vi "Measurement.vi"(0 "Position":T7(array[cluster]) {"Z" format="%.1f"; "Y" format="%.1f"; "X" format="%.1f"}, 1 "setup":T8=enum."Show Setup", 2 "Post Process":T5, 4 "File":T9, 5 "Results file":path, 7 "Raw data file":path, 11 "Setup filename":string) -> (14 "2nd plot":cluster{"Xo":dbl, "Delta X":dbl, dbl[]}[](graph), 19 "Status Out":T4)   [LabVIEW 2010]
uses:
  Anemometry Sub Vis/Controls/Save_Data.ctl
  Anemometry Sub Vis/Controls/Setup.ctl
  Anemometry Sub Vis/Controls/Graph_Type.ctl
  Anemometry Sub Vis/Controls/Post_Process.ctl
  Anemometry Sub Vis/Gen Trav/Multi_Run_Status.ctl
  Anemometry Sub Vis/Controls/Board_Types.ctl
  Anemometry Sub Vis/Controls/Block_start_and_end.ctl
  ADAM Client/Sub VIs/ADAM Controls/Traverse_Level_State.ctl
  Anemometry Sub Vis/Globals/Trav_pos_global.vi
  Anemometry Sub Vis/Globals/Meas_global.vi
  Anemometry Sub Vis/Acquisition/PWA/PWAtasksGLOBAL.vi
  Anemometry Sub Vis/Globals/Preference_global.vi
  Anemometry Sub Vis/Globals/LDA_meas_global_1.vi
  Anemometry Sub Vis/Globals/Dynamic_call_global.ph.vi
  Anemometry Sub Vis/Globals/LDA_meas_global_2.vi
  Anemometry Sub Vis/Globals/Constants_global.vi
  Anemometry Sub Vis/Globals/Plug_in_data_global.vi
panel:
  in  "PP next block":bool
  out "Pause message":string
  out "Statistics":string[][](table)
  in  "Tab Control":T1(tab)
  out "Measurement time (min)":dbl=6.0 format="%.2f"
  in  "No of bins":i32=80
  in  "Show Smoth":bool=TRUE
  in  "Second Graph":T3={"Plot 1"=2, "Plot 2"=1, "Save graph"=0, "Plot Type"=enum."Vel histogram"} {"Save graph" items=["Do not save plot", "Save plot"]; "Plot 2" items=["Nothing", "LDA (U)", "LDA (W)", "HW (HW) LDA Sync", "HW (HW)", "RV (WT)", "RV (WT2)"]; "Plot 1" items=["Nothing", "LDA (U)", "LDA (W)", "HW (HW) LDA Sync", "HW (HW)", "RV (WT)", "RV (WT2)"]}
  in  "First Graph":T3={"Plot 1"=1, "Plot 2"=2, "Save graph"=0, "Plot Type"=enum."Velocity trace"} {"Save graph" items=["Do not save plot", "Save plot"]; "Plot 2" items=["Nothing", "LDA (U)", "LDA (W)", "HW (HW) LDA Sync", "HW (HW)", "RV (WT)", "RV (WT2)"]; "Plot 1" items=["Nothing", "LDA (U)", "LDA (W)", "HW (HW) LDA Sync", "HW (HW)", "RV (WT)", "RV (WT2)"]}
  out "First plot":cluster{"Xo":dbl, "Delta X":dbl, dbl[]}[](graph)
  in  "Comments":string
  out "BSA Diagnostic info":string[][](table)
  out "uv":dbl[][](graph)=[[-0.041806189081711534, -0.046435429052714985, -0.04035660097427599, -0.042187605126076694, -0.042052555599004206]]
  out "u^4":dbl[][](graph)
  out "u^3":dbl[][](graph)
  out "u^2":dbl[][](graph)=[[0.09743628875280319, 0.10575821456272283, 0.10126262927293661, 0.09890442087602569, 0.1022948212436432]]
  out "U":dbl[][](graph)=[[0.8295029456391334, 0.8915896983798417, 0.8415763502225625, 0.8394746126219594, 0.8466062785395404]]
  in  "Block average display control":cluster{"Name":string, "Include":bool}[](array[cluster])=[{"Name"="FF (C)", "Include"=FALSE}]
  out "Array U":dbl[][](array[numeric]) format="%.2e"
  out "Array u^2":dbl[][](array[numeric]) format="%.2e"
  out "Actual Sampling freq":dbl=100.0 format="%.1f"
  in  "Desired Sampling freq (Hz)":dbl=100.0 format="%.1f"
  in  "Correlate?":T6(ring)
  out "Current Block No":i32=5
  in  "Pause":bool
  in  "No of Blocks":i32=5
  in  "stop":bool
  in  "No of samples":i32=1000 min=0 step=1
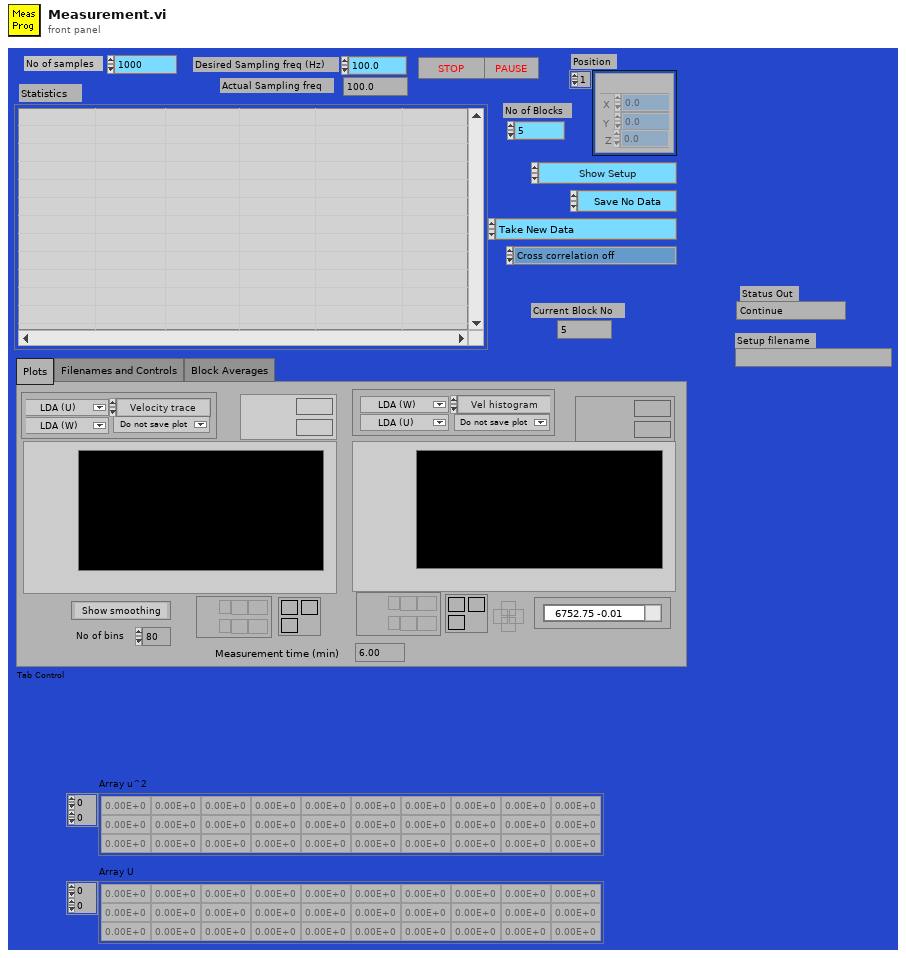
[diagram p1: front panel]
types:
  T1 = enum32{"Plots", "Filenames and Controls", "Block Averages"}
  T2 = typedef "Graph_Type.ctl" = enum16{"Show no graph", "Voltage trace", "Velocity trace", "Vel histogram", "Spectrum", "f.E(f) v Log f", "Auto-Corr"}
  T3 = cluster{"Plot 1":u16, "Plot 2":u16, "Save graph":u16, "Plot Type":T2}
  T4 = typedef "Multi_Run_Status.ctl" = enum16{"Continue", "Jump to Next Point", "Jump to Next Row", "Jump To Fall Back", "Terminate Run"}
  T5 = typedef "Post_Process.ctl" = enum16{"Take New Data", "Post Process Raw Data File"}
  T6 = enum16{"Cross correlation off", "Show correlation panel", "Correlate without activating panel"}
  T7 = cluster{"Name":string, "X":dbl, "Y":dbl, "Z":dbl}[]
  T8 = typedef "Setup.ctl" = enum16{"Run Program", "Show Setup", "Save Current Setup", "Setup Front Panel"}
  T9 = typedef "Save_Data.ctl" = enum16{"Save No Data", "Save Data"}
  T10 = enum32{"Bad", "Idle", "Run top level", "Running"}
  T11 = enum16{"Velocity", "Transit time", "Arrival time"}
  T12 = enum16{"Save no data", "Save data in new files", "Save data in existing files"}
  T13 = typedef "Board_Types.ctl" = enum16{"Simulate", "NB-MIO-16H", "PCI-MIO-16E", "6000E Series", "USB-92xx", "ADC488", "Lab-NB", "NB-DIO-24", "NI-DAQmx", "Local ADAM", "Server Channels"}
  T14 = typedef "Block_start_and_end.ctl" = cluster{"Started":dbl, "Ended":dbl, "Analogue Frequency Hz":dbl}
  T15 = typedef "Traverse_Level_State.ctl" = enum16{"Running", "Complete"}
  T16 = typedef "Traverse_cluster.ctl" = cluster{"Start X":dbl, "Start Y":dbl, "Start Z":dbl, "End X":dbl, "End Y":dbl, "End Z":dbl, "No. of pts.":i32, "Spacing":T17, "Filename":path, "Tunnel Speed":dbl, "Averaging time (min)":dbl, "Extra Commands":string, "Specific Arguments":string, "Emission Rate (l/min)":dbl, "Trace Gas Concentration (%)":dbl, "Density Ratio":string, "Comments":string, "Row No":i32, "Row Type Selector":T18, "Completion time":string, "Row Duration (mins)":dbl, "No. of Valid pts.":i32, "Meas Setup File":string}
  T17 = typedef "Spacing.ctl" = enum16{"Linear", "Log", "Gauss", "Specified", "N/A"}
  T18 = typedef "Multi_run_mode.ctl" = enum16{"Move Traverse Only", "Set Tunnel Speed Only", "Set Source Only", "Set Measurement Conditions", "Single Measurement", "Vertical Profile", "Lateral Profile", "Longitudinal Profile", "Explore Volume", "Multi-Axis Profile", "Auto Calibrate", "Meas Fast FID Bkgnd", "Check Beam Power", "Scanning Valve Measurement", "Run VI Named:", "Set ADAM Ch", "Wait (minutes)", "Send Message", "Synchronize With:", "Fall Back to this Row", "Turn Off Row Repeating", "Blank Row"}
  T19 = typedef "Analysis_info_cluster.ctl" = cluster{"Colour":u32, "Inst type":T20, "Inst name":string, "Symbol":string, "Code name":string, "Extra Info":string, "Inst Array":T21, "Index":i32, "Voltage Index":i32, "Extra Titles":string[], "Extra Values":string[]}
  T20 = typedef "Inst_type.ctl" = enum16{"Propeller anemometer", "Raw voltage", "Pressure Transducer", "Pitot-static tube", "Preston tube", "Hot wire", "Cross wire 1", "Cross wire 2", "Generic Linear", "Generic Polynomial", "Generic BackPoly", "Fast FID", "Thermocouple", "Cold wire", "Pulsed Wire", "LDA Vel", "LDA Tran time", "LDA Arr time"}
  T21 = typedef "Instrument_Array.ctl" = enum16{"PWA", "LDA", "Analogue"}
  T22 = enum16{"Velocity", "Transit time", "Arrival time"}[]
  T23 = typedef "BSA_Type.ctl" = enum16{"57N11", "BSA F60"}
  T24 = typedef "BSA_info_Cluster.ctl" = cluster{"GPIB Address":string, "No of Check Bytes":i32, "Extra Info":string, "COLOUR":u32, "Wavelength (nm)":dbl}
  T25 = typedef "Ch_and_Spans.ctl" = cluster{"high limit (10V)":sgl, "low limit (-10V)":sgl, "Ch No":i16, "Var name":string, "Use Latest Calib":bool}
  T26 = typedef "Velocity_cluster.ctl" = cluster{"Name":string, "U":dbl, "u^2":dbl, "u^3/(u^2)^(1.5)":dbl, "u^4/(u^2)^2 -3":dbl, "% u'/U":dbl, "Mean % Err":dbl, "u^4":dbl}
  T27 = typedef "Analysis_type_cluster.ctl" = cluster{"Analysis type":T28, "Indicies":i32[], "Name":string, "Inst Array":T21, "Info index":i32}
  T28 = typedef "Analysis_type_Enum.ctl" = enum16{"Slow Response", "Fast Response", "Weighted Fast Response", "Fast FID", "Weighted Fast FID", "Cross Wire", "Weighted Cross Wire", "Weighted LDA"}
  T29 = cluster{"Insts for plotting[0]":u16, "Insts for plotting[1]":u16}
  T30 = typedef "PWA_Data.ctl" = enum16{"No PWA Data", "One Ch PWA"}
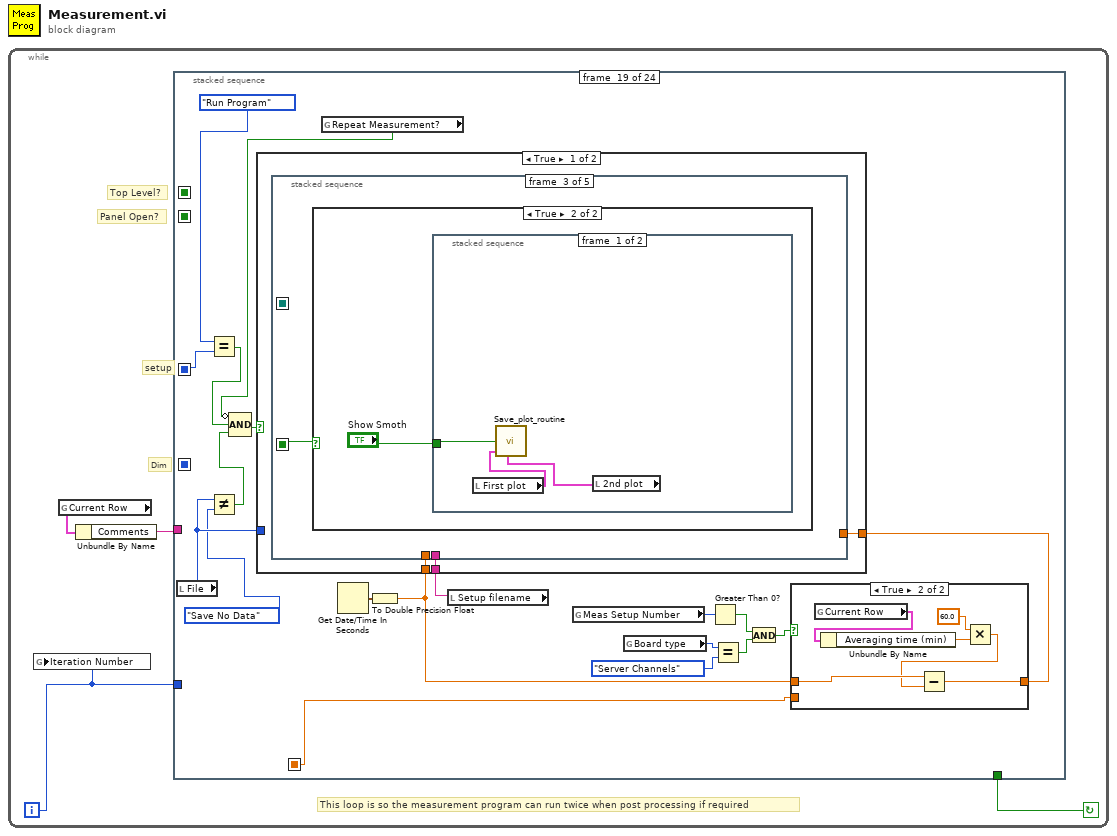
[diagram p0: block diagram]
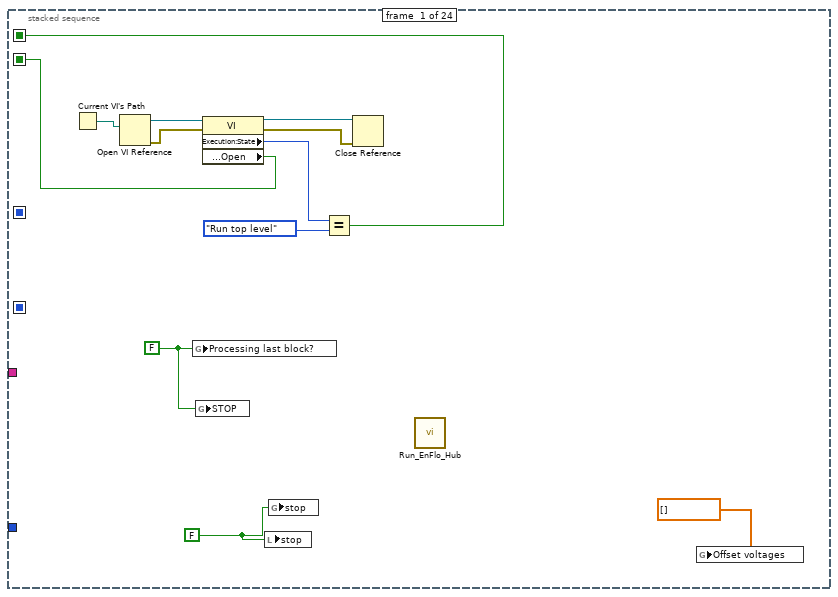
[diagram p2: hidden frame]
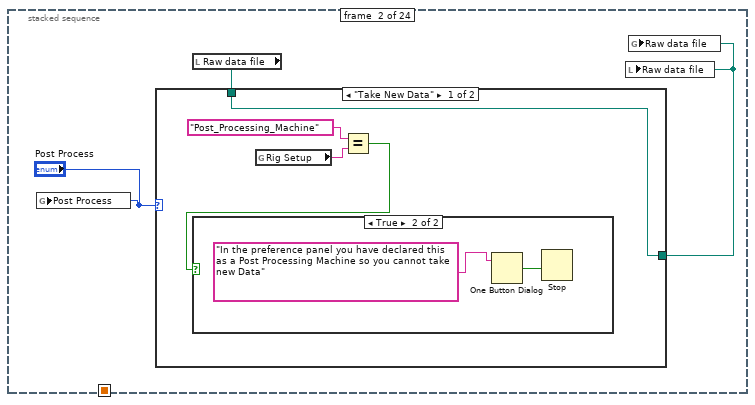
[diagram p3: hidden frame]
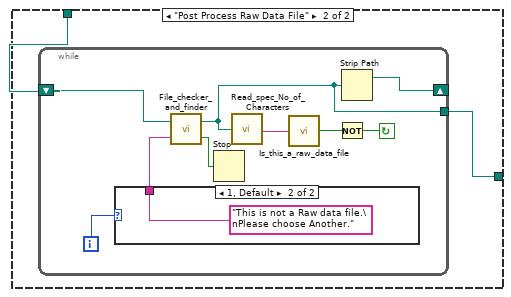
[diagram p5: hidden frame]
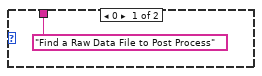
[diagram p6: hidden frame]
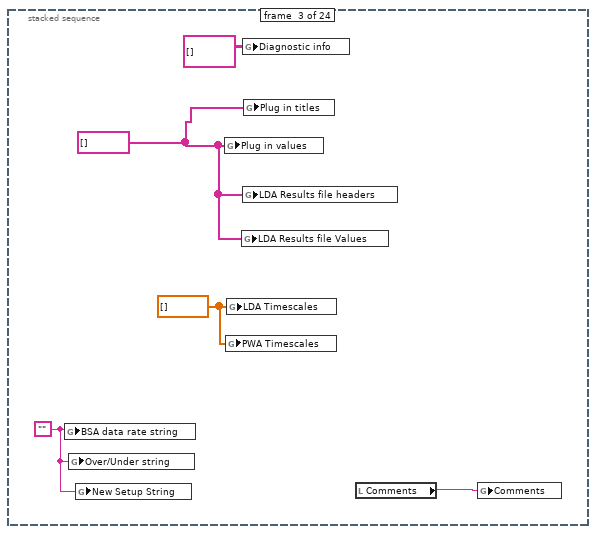
[diagram p7: hidden frame]
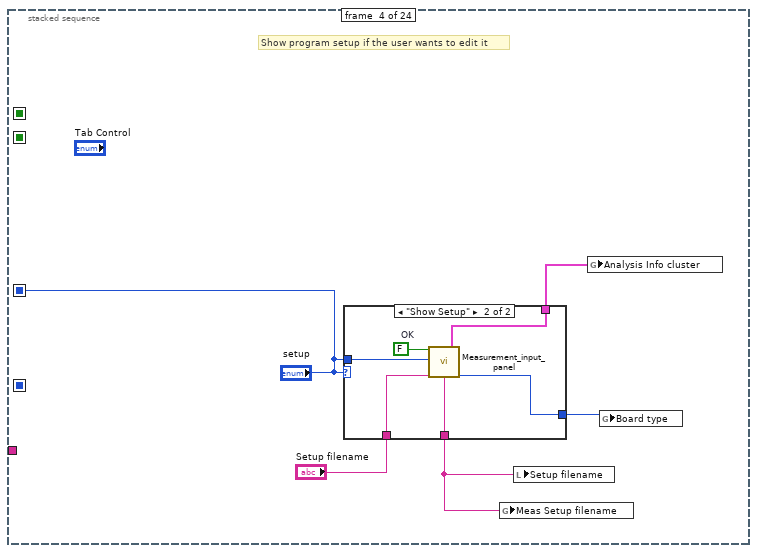
[diagram p8: hidden frame]
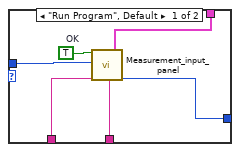
[diagram p9: hidden frame]
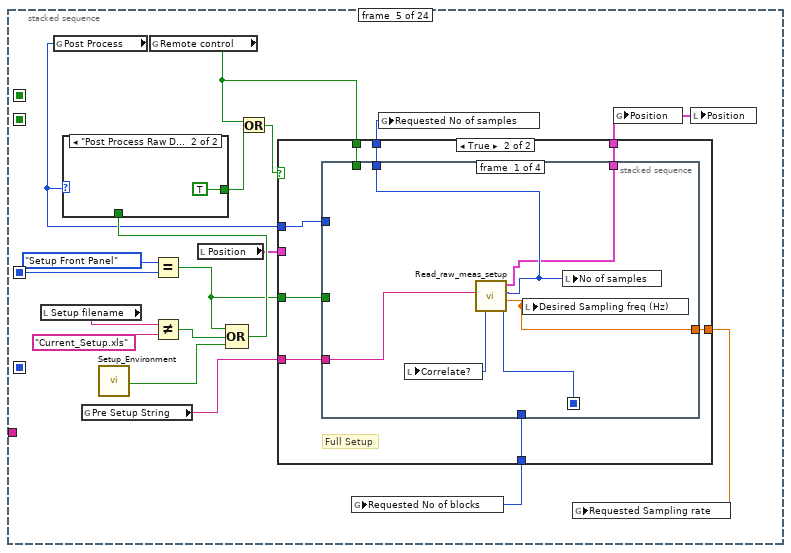
[diagram p10: hidden frame]
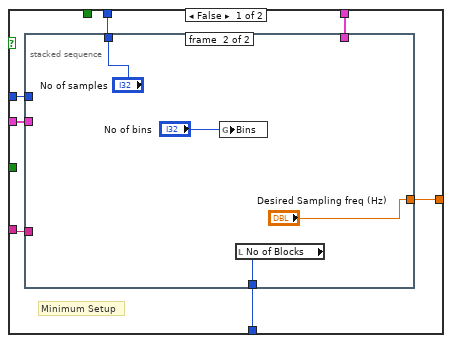
[diagram p12: hidden frame]
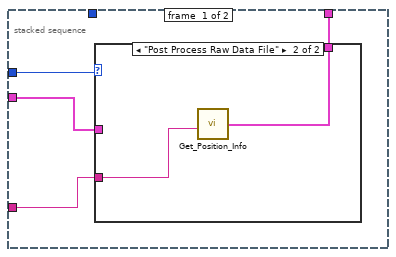
[diagram p13: hidden frame]
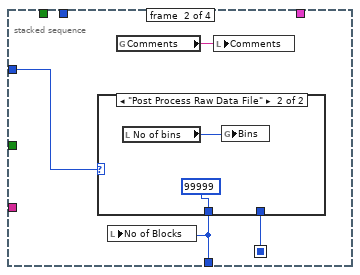
[diagram p15: hidden frame]
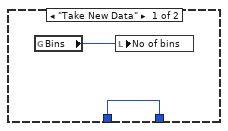
[diagram p16: hidden frame]
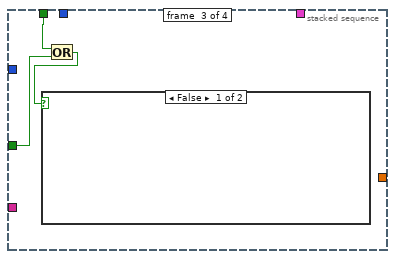
[diagram p17: hidden frame]
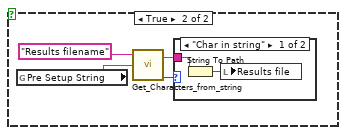
[diagram p18: hidden frame]
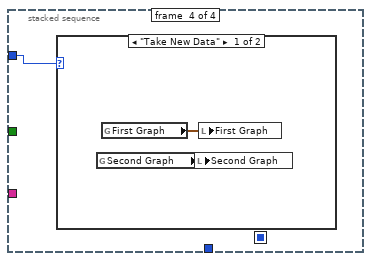
[diagram p20: hidden frame]
diagram:
  n1 = while {
    i -> [w1]
    stop <- w2 continue-if-true
    # "This loop is so the measurement program can run twice when post processing if required"
    # "Panel Open?"
    # "Top Level?"
    # "setup"
    # "Dim"
    n2 = global write "Meas_global.vi" "Iteration Number"(w1) -> ()
    n3 = global read "Trav_pos_global.vi" "Current Row"() -> (w3:T16)
    n4 = Unbundle By Name(w3) -> ("Comments"=w4:string)
    n5 = stacked-sequence {
      seq-local: [_ _ _ _ _ _ _ _ w186 _ _ _ _ _ _ _ _ _ _ _ _ _ _ _] -> [_ _ _ _ _ _ _ _ _ _ _ _ _ _ _ _ _ w631 _ _ _ _ _ _]
      seq-local: [_ _ _ "setup" _ _ _ _ _ _ _ _ _ _ _ _ _ _ _ _ _ _ _ _] -> [_ _ _ _ w70 _ _ _ w178 w263 _ _ _ _ w523 w561 w569 w632 w940 w1016 w1044 _ _ w1119]
      seq-local: [_ _ _ _ _ _ _ _ _ _ _ _ _ _ _ _ w564 _ _ _ _ _ _ _] -> [_ _ _ _ _ _ _ _ _ _ _ _ _ _ _ _ _ w630 w923 _ _ _ _ _]
      seq-local: [w6 _ _ _ _ _ _ _ _ _ _ _ _ _ _ _ _ _ _ _ _ _ _ _] -> [_ _ _ _ _ _ _ _ _ w243 _ _ _ _ w519 _ _ w629 _ _ _ _ _ _]
      seq-local: [w5 _ _ _ _ _ _ _ _ _ _ _ _ _ _ _ _ _ _ _ _ _ _ _] -> [_ _ _ _ _ _ _ _ _ _ _ _ w363 _ _ _ _ _ _ _ _ _ _ _]
      tunnel: w4 -> [_ _ _ _ _ _ _ w171 _ _ _ _ _ _ _ _ _ _ _ _ _ _ w1087 _]
      tunnel: w1 -> [_ _ _ _ _ _ _ _ _ _ _ _ _ _ _ _ _ _ _ _ _ _ w1082 _]
      tunnel: [_ _ _ _ _ _ _ _ _ _ _ _ _ _ _ _ _ _ _ _ _ _ w1081 _] -> w2
      frame #0 {
        w14 = FALSE ("Processing last block?")
        w15 = FALSE ("stop")
        n6 = Current VI's Path() -> (path=w7:path)
        n7 = Open VI Reference(vi path=w7) -> (vi reference=w8:refnum<vi>, error out=w9:errorcluster)  [unwired: 1 in, 4 out]
        n8 = global write "Meas_global.vi" "Processing last block?"(w14) -> ()
        n9 = global write "PWAtasksGLOBAL.vi" "STOP"(w14) -> ()
        n10 = property class="VI"(reference=w8, error in=w9) -> (reference out=w10:refnum<vi>, error out=w11:errorcluster, "Execution:State"=w12:T10, "Front Panel.Open"=w5:bool)
        n11 = local write "stop"(w15) -> ()
        n12 = global write "Meas_global.vi" "stop"(w15) -> ()
        n13 = Equal?(x=w12, y=T10."Run top level" ("Exec.State")) -> (x = y?=w6:bool)
        n14 = Close Reference(reference=w10, error in (no error)=w11) -> ()  [unwired: 1 out]
        n15 = call "Run_EnFlo_Hub.vi"() -> ()  [unwired: 8 out]
        n16 = global write "Meas_global.vi" "Offset voltages"(dbl[] [] ("Offset voltages used")) -> ()
      }
      frame #1 {
        n17 = global write "Meas_global.vi" "Post Process"("Post Process") -> ()
        n18 = local read "Raw data file"() -> (w19:path)
        n19 = case shown="\"Take New Data\"" "Post Process" {
          tunnel: [w23 w27] -> w18
          tunnel: w19 -> [w23 w26]
          frame "Take New Data" {
            n20 = global read "Preference_global.vi" "Rig Setup"() -> (w22:string)
            n21 = Equal?(x="Post_Processing_Machine" ("Rig Setup"), y=w22) -> (x = y?=w20:bool)
            n22 = case shown="True" w20 {
              frame False {
              }
              frame True {
                n23 = One Button Dialog(message="In the preference panel you have declared this as a Post Processing Machine so you cannot take new Data") -> (true=w24:bool)  [unwired: 1 in]
                n24 = Stop(stop? (T)=w24) -> ()
              }
            }
          }
          frame "Post Process Raw Data File" {
            n25 = while {
              tunnel: [w29] -> w27
              shift-left: w26 -> [w31]
              shift-right: [w30] -> _
              i -> [w32]
              stop <- w33 continue-if-true
              n26 = case shown="1, Default" w32 {
                tunnel: ["Find a Raw Data File to Post Process" ("Promp if not found") "This is not a Raw data file.\nPlease choose Another." ("Promp if not found")] -> w36
                frame 0 {
                }
                frame 1, Default {
                }
              }
              n27 = call "File_checker_and_finder.vi"("Promp if not found"=w36, "Filename In"=w31) -> ("cancelled"=w28:bool, "Filename Out"=w29:path)
              n28 = Stop(stop? (T)=w28) -> ()
              n29 = call "Read_spec_No_of_Characters.vi"("Filename"=w29) -> ("character string"=w35:string)  [unwired: 1 out]
              n30 = call "Is_this_a_raw_data_file.vi"("character string"=w35) -> ("Raw Dat File?"=w34:bool)  [unwired: 2 out]
              n31 = Not(x=w34) -> (.not. x?=w33:bool)
              n32 = Strip Path(path=w29) -> (stripped path=w30:path)  [unwired: 1 out]
            }
          }
        }
        n33 = local write "Raw data file"(w18) -> ()
        n34 = global write "Meas_global.vi" "Raw data file"(w18) -> ()
      }
      frame #2 {
        w41 = dbl[] [] ("LDA Timescales")
        w40 = string[] [] ("Plug in values")
        w43 = ""
        n35 = global write "Meas_global.vi" "BSA data rate string"(w43) -> ()
        n36 = global write "Meas_global.vi" "Over/Under string"(w43) -> ()
        n37 = global write "Meas_global.vi" "New Setup String"(w43) -> ()
        n38 = global write "Dynamic_call_global.ph.vi" "Plug in values"(w40) -> ()
        n39 = global write "PWAtasksGLOBAL.vi" "PWA Timescales"(w41) -> ()
        n40 = global write "LDA_meas_global_1.vi" "LDA Timescales"(w41) -> ()
        n41 = global write "LDA_meas_global_1.vi" "LDA Results file Values"(w40) -> ()
        n42 = global write "Meas_global.vi" "Diagnostic info"(string[][] [] ("Diagnostic info")) -> ()
        n43 = global write "LDA_meas_global_1.vi" "LDA Results file headers"(w40) -> ()
        n44 = global write "Dynamic_call_global.ph.vi" "Plug in titles"(w40) -> ()
        n45 = local read "Comments"() -> (w42:string)
        n46 = global write "Meas_global.vi" "Comments"(w42) -> ()
      }
      frame #3 {
        # "Show program setup if the user wants to edit it"
        n47 = case shown="\"Show Setup\"" "setup" {
          tunnel: [w53 w59] -> w48
          tunnel: [w52 w58] -> w47
          tunnel: "Setup filename" -> [w51 w57]
          tunnel: [w50 w56] -> w44
          tunnel: "setup" -> [w49 w55]
          frame "Run Program", Default {
            w54 = TRUE  # OK
            n48 = call "Measurement_input_panel.vi"("OK"=w54, "setup"=w49, "Setup filename"=w51) -> ("Setup filename out"=w50:string, "Analysis Info cluster"=w53:T19[], "Board type"=w52:T13)  [unwired: 14 out]
          }
          frame "Show Setup" {
            w60 = FALSE  # OK
            n49 = call "Measurement_input_panel.vi"("OK"=w60, "setup"=w55, "Setup filename"=w57) -> ("Setup filename out"=w56:string, "Analysis Info cluster"=w59:T19[], "Board type"=w58:T13)  [unwired: 14 out]
          }
        }
        n50 = global write "Meas_global.vi" "Meas Setup filename"(w44) -> ()
        n51 = local write "Setup filename"(w44) -> ()
        n52 = global write "Meas_global.vi" "Analysis Info cluster"(w48) -> ()
        n53 = global write "Meas_global.vi" "Board type"(w47) -> ()
      }
      frame #4 {
        n54 = local read "Setup filename"() -> (w74:string)
        n55 = global read "Meas_global.vi" "Post Process"() -> (w69:T5)
        n56 = global read "Meas_global.vi" "Pre Setup String"() -> (w65:string)
        n57 = call "Setup_Environment.vi"() -> ("First Time"=w66:bool)  [unwired: 1 in]
        n58 = global read "Meas_global.vi" "Remote control"() -> (w62:bool)
        n59 = Equal?(x=Setup."Setup Front Panel" ("setup"), y=w70) -> (x = y?=w61:bool)
        n60 = Not Equal?(x=w74, y="Current_Setup.xls" ("Setup filename")) -> (x != y?=w72:bool)
        n61 = local read "Position"() -> (w63:T7)
        n62 = Compound Arithmetic op=OR(w61, w72, w66) -> (w71:bool)
        n63 = case shown="\"Post Process Raw Data File\"" w69 {
          tunnel: [w79 TRUE] -> w78
          tunnel: w71 -> [w79 _]
          frame "Take New Data" {
          }
          frame "Post Process Raw Data File" {
          }
        }
        n64 = Or(x=w62, y=w78) -> (x .or. y?=w77:bool)
        n65 = case shown="True" w77 {
          tunnel: w69 -> [w83 w106]
          tunnel: [w87 w105] -> w67
          tunnel: [w86 w100] -> w76
          tunnel: [w85 w104] -> w75
          tunnel: [w84 w103] -> w64
          tunnel: w65 -> [w82 w102]
          tunnel: w63 -> [w81 _]
          tunnel: w62 -> [_ w101]
          tunnel: w61 -> [_ w99]
          frame False {
            # "Minimum Setup"
            n66 = stacked-sequence {
              tunnel: [_ "Desired Sampling freq (Hz)"] -> w87
              tunnel: [_ w97] -> w86
              tunnel: [_ "No of samples"] -> w85
              tunnel: [w90 _] -> w84
              tunnel: w83 -> [w91 _]
              tunnel: w82 -> [w89 _]
              tunnel: w81 -> [w88 _]
              frame #0 {
                n67 = case shown="\"Post Process Raw Data File\"" w91 {
                  tunnel: [w92 w93] -> w90
                  tunnel: w88 -> [w92 _]
                  tunnel: w89 -> [_ w94]
                  frame "Take New Data" {
                  }
                  frame "Post Process Raw Data File" {
                    n68 = call "Get_Position_Info.vi"("Input string"=w94) -> ("Position"=w93:T7)
                  }
                }
              }
              frame #1 {
                n69 = global write "Meas_global.vi" "Bins"("No of bins") -> ()
                n70 = local read "No of Blocks"() -> (w97:i32)
              }
            }
          }
          frame True {
            # "Full Setup"
            n71 = stacked-sequence {
              seq-local: [w109 _ _ _] -> [_ w114 _ _]
              tunnel: w106 -> [_ w115 _ w130]
              tunnel: [w112 _ _ _] -> w105
              tunnel: [w111 _ _ _] -> w104
              tunnel: [w107 _ _ _] -> w103
              tunnel: w102 -> [w110 _ _ _]
              tunnel: w101 -> [_ _ w123 _]
              tunnel: [_ w113 _ _] -> w100
              tunnel: w99 -> [_ _ w122 _]
              frame #0 {
                n72 = call "Read_raw_meas_setup.vi"("Setup file string"=w110) -> ("No of Blocks"=w109:i32, "Sampling freq (Hz)"=w112:dbl, "No of samples"=w111:i32, "Position"=w107:T7, "Correlate?"=w108:T6)  [unwired: 4 out]
                n73 = local write "Correlate?"(w108) -> ()
                n74 = local write "Desired Sampling freq (Hz)"(w112) -> ()
                n75 = local write "No of samples"(w111) -> ()
              }
              frame #1 {
                n76 = case shown="\"Post Process Raw Data File\"" w115 {
                  tunnel: [w118 99999 ("No of Blocks")] -> w113
                  tunnel: w114 -> [w118 _]
                  frame "Take New Data" {
                    n77 = global read "Meas_global.vi" "Bins"() -> (w117:i32)
                    n78 = local write "No of bins"(w117) -> ()
                  }
                  frame "Post Process Raw Data File" {
                    n79 = local read "No of bins"() -> (w119:i32)
                    n80 = global write "Meas_global.vi" "Bins"(w119) -> ()
                  }
                }
                n81 = local write "No of Blocks"(w113) -> ()
                n82 = global read "Meas_global.vi" "Comments"() -> (w116:string)
                n83 = local write "Comments"(w116) -> ()
              }
              frame #2 {
                n84 = Or(x=w123, y=w122) -> (x .or. y?=w121:bool)
                n85 = case shown="False" w121 {
                  frame False {
                  }
                  frame True {
                    n86 = global read "Meas_global.vi" "Pre Setup String"() -> (w124:string)
                    n87 = call "Get_Characters_from_string.vi"("Input string"=w124, "Variable name"="Results filename") -> ("Status"=w127:enum16{"Char in string", "Char not in string"}, "Value"=w126:string)  [unwired: 1 in]
                    n88 = case shown="\"Char in string\"" w127 {
                      tunnel: w126 -> [w129 _]
                      frame "Char in string" {
                        n89 = String To Path(string=w129) -> (path=w128:path)
                        n90 = local write "Results file"(w128) -> ()
                      }
                      frame "Char not in string" {
                      }
                    }
                  }
                }
              }
              frame #3 {
                n91 = case shown="\"Take New Data\"" w130 {
                  frame "Take New Data" {
                    n92 = global read "Meas_global.vi" "Second Graph"() -> (w131:T3)
                    n93 = global read "Meas_global.vi" "First Graph"() -> (w132:T3)
                    n94 = local write "Second Graph"(w131) -> ()
                    n95 = local write "First Graph"(w132) -> ()
                  }
                  frame "Post Process Raw Data File" {
                  }
                }
              }
            }
          }
        }
        n96 = global write "Meas_global.vi" "Requested No of blocks"(w76) -> ()
        n97 = global write "Meas_global.vi" "Requested No of samples"(w75) -> ()
        n98 = global write "Meas_global.vi" "Requested Sampling rate"(w67) -> ()
        n99 = global write "Meas_global.vi" "Position"(w64) -> ()
        n100 = local write "Position"(w64) -> ()
      }
      frame #5 {
        n101 = global read "Meas_global.vi" "Post Process"() -> (w133:T5)
        n102 = case shown="\"Post Process Raw Data File\"" w133 {
          tunnel: [w136 w137] -> w134
          frame "Take New Data" {
            n103 = Get Date/Time In Seconds() -> (seconds since 1Jan1904=w135:timestamp)
            n104 = To Double Precision Float(number=w135) -> (double precision float=w136:dbl)
          }
          frame "Post Process Raw Data File" {
            n105 = global read "Meas_global.vi" "Pre Setup String"() -> (w140:string)
            n106 = call "Get_Characters_from_string.vi"("Input string"=w140, "Variable name"="Seconds since 1/1/04") -> ("Value"=w138:string)  [unwired: 1 in, 1 out]
            n107 = Fract/Exp String To Number(string=w138) -> (number=w137:dbl)  [unwired: 4 out]
          }
        }
        n108 = global write "Meas_global.vi" "Time Data was Aquired"(w134) -> ()
      }
      frame #6 {
        n109 = global read "Dynamic_call_global.ph.vi" "Initial Plug Ins"() -> (w142:string[])
        n110 = global read "Dynamic_call_global.ph.vi" "Initial Plug Ins Extra"() -> (w143:string[])
        n111 = Build Array (concatenate)(w143, w142) -> (w141:string[])
        n112 = Array Size(array=w141) -> (size(s)=w145:i32)
        n113 = Greater Than 0?(x=w145) -> (x > 0?=w144:bool)
        n114 = case shown="True" w144 {
          tunnel: w141 -> [_ w146]
          frame False {
          }
          frame True {
            n115 = stacked-sequence {
              tunnel: w146 -> [w148 _]
              frame #0 {
                n116 = global read "Meas_global.vi" "Post Process"() -> (w150:T5)
                n117 = call "Plug_in_Directories.vi"() -> ("Initial"=w147:path)  [unwired: 3 out]
                n118 = Equal?(x=w150, y=Post_Process."Post Process Raw Data File" ("Post Process")) -> (x = y?=w149:bool)
                n119 = for {
                  tunnel: w149 -> [w156]
                  tunnel: w148 -> [w153] mode=indexing
                  tunnel: w147 -> [w152]
                  w163 = FALSE  # Dialog Box (T)
                  n120 = Build Path(base path=w152, name or relative path=w153) -> (appended path=w154:path)
                  n121 = Open VI Reference(vi path=w154) -> (vi reference=w161:refnum<vi>, error out=w160:errorcluster)  [unwired: 2 in, 3 out]
                  n122 = property class="VI"(reference=w161, error in=w160, "Front Panel Window:Open"=TRUE ("Wait until done")) -> (reference out=w159:refnum<vi>, error out=w158:errorcluster)
                  n123 = invoke class="VI" method="Run VI"(reference=w159, error in=w158, "Wait until done"=w156, "Auto Dispose Ref"=FALSE) -> (reference out=w166:refnum<vi>, error out=w165:errorcluster)  [unwired: 1 in, 3 out]
                  n124 = Close Reference(reference=w166, error in (no error)=w165) -> (error out=w164:errorcluster)
                  n125 = call "EnFlo_Error_Handler.vi"("error in (no error)"=w164, "Error Type"="Launching Initial Plug In", "Dialog Box (T)"=w163) -> ()  [unwired: 3 out]
                }
              }
              frame #1 {
                n126 = global read "Meas_global.vi" "Requested No of blocks"() -> (w168:i32)
                n127 = global read "Meas_global.vi" "Comments"() -> (w167:string)
                n128 = local write "Comments"(w167) -> ()
                n129 = local write "No of Blocks"(w168) -> ()
              }
            }
          }
        }
      }
      frame #7 {
        n130 = local read "Comments"() -> (w172:string)
        n131 = Concatenate Strings(w171, w172) -> (w170:string)
        n132 = call "Text_without_format.vi"("Input string"=w170) -> ("Output string"=w169:string)
        n133 = local write "Comments"(w169) -> ()
        n134 = global write "Meas_global.vi" "Comments"(w169) -> ()
      }
      frame #8 {
        n135 = global read "Meas_global.vi" "dimensions"() -> (w186:enum16{"1D", "2D"})
        n136 = global read "Meas_global.vi" "Post Process"() -> (w185:T5)
        n137 = global read "Meas_global.vi" "LDA data"() -> (w183:enum16{"No LDA data", "Take LDA data"})
        n138 = Equal?(x=Setup."Run Program" ("setup"), y=w178) -> (x = y?=w181:bool)
        n139 = Equal?(x=w178, y=Setup."Show Setup" ("setup")) -> (x = y?=w173:bool)
        n140 = Equal?(x=w183, y=enum16{"No LDA data", "Take LDA data"}."Take LDA data" ("LDA data")) -> (x = y?=w176:bool)
        n141 = Or(x=w181, y=w173) -> (x .or. y?=w175:bool)
        n142 = Equal?(x=w185, y=Post_Process."Take New Data" ("Post Process")) -> (x = y?=w177:bool)
        n143 = Compound Arithmetic op=AND(w175, w176, w177) -> (w174:bool)
        n144 = case shown="True" w174 {
          tunnel: w186 -> [_ w195]
          tunnel: w178 -> [_ w194]
          tunnel: w173 -> [_ w192]
          frame False {
            n145 = global write "LDA_meas_global_1.vi" "Number of measured quantities"(3 ("Number of measured quantities")) -> ()
            n146 = Build Array(T11."Velocity", T11."Transit time", T11."Arrival time") -> (w187:T22)
            n147 = global write "LDA_meas_global_2.vi" "data type"(w187) -> ()
            n148 = global write "LDA_meas_global_1.vi" "data type"(w187) -> ()
          }
          frame True {
            n149 = global read "LDA_meas_global_1.vi" "BSA Type"() -> (w193:T23)
            n150 = case shown="\"BSA F60\"" w193 {
              tunnel: w195 -> [w197 _]
              tunnel: w194 -> [w196 _]
              tunnel: w192 -> [_ w233]
              frame "57N11" {
                n151 = stacked-sequence {
                  tunnel: w197 -> [w200 w226]
                  tunnel: w196 -> [w199 _]
                  frame #0 {
                    n152 = global read "Meas_global.vi" "Remote control"() -> (w198:bool)
                    n153 = case shown="\"2D\"" w200 {
                      tunnel: w199 -> [w202 w215]
                      tunnel: w198 -> [w201 w214]
                      frame "2D" {
                        n154 = while {
                          tunnel: w201 -> [w203]
                          tunnel: w202 -> [w204]
                          stop <- w205 continue-if-true
                          n155 = stacked-sequence {
                            tunnel: [_ _ w211] -> w205
                            tunnel: w204 -> [w206 w208 _]
                            tunnel: w203 -> [_ _ w210]
                            frame #0 {
                              w207 = "1"  # BSA Number
                              n156 = call "Control_BSA_setup.vi"("setup"=w206, "BSA number"=w207) -> ()  [unwired: 14 out]
                            }
                            frame #1 {
                              w209 = "2"  # BSA Number
                              n157 = call "Control_BSA_setup.vi"("setup"=w208, "BSA number"=w209) -> ()  [unwired: 14 out]
                            }
                            frame #2 {
                              n158 = case shown="False" w210 {
                                tunnel: [w212 FALSE ("ok")] -> w211
                                frame False {
                                n159 = call "BSA_setup_check.vi"() -> ("ok"=w212:bool)
                                }
                                frame True {
                                }
                              }
                            }
                          }
                        }
                      }
                      frame "1D" {
                        n160 = stacked-sequence {
                          tunnel: w215 -> [w216 _]
                          tunnel: w214 -> [_ _]
                          frame #0 {
                            w217 = "1"  # BSA Number
                            n161 = call "Control_BSA_setup.vi"("setup"=w216, "BSA number"=w217) -> ()  [unwired: 14 out]
                          }
                          frame #1 {
                            n162 = global read "LDA_meas_global_2.vi" "BSA2 info"() -> (w218:T24)
                            n163 = Unbundle By Name(w218) -> ("GPIB Address"=w219:string)
                            n164 = call "Set_BSA_Coincidence.vi"("GPIB address"=w219, "Set Coincidence"=enum16{"Slave", "Master", "Private"}."Slave") -> ()  [unwired: 1 in, 5 out]
                          }
                        }
                      }
                    }
                  }
                  frame #1 {
                    n165 = global read "Meas_global.vi" "Remote control"() -> (w224:bool)
                    n166 = Equal?(x=w226, y=enum16{"1D", "2D"}."2D" ("dimensions")) -> (x = y?=w222:bool)
                    n167 = Not(x=w224) -> (.not. x?=w223:bool)
                    n168 = And(x=w223, y=w222) -> (x .and. y?=w221:bool)
                    n169 = case shown="True" w221 {
                      frame False {
                      }
                      frame True {
                        n170 = global read "LDA_meas_global_1.vi" "BSA1 info"() -> (w228:T24)
                        n171 = global read "LDA_meas_global_2.vi" "BSA2 info"() -> (w229:T24)
                        n172 = Build Array(w228, w229) -> (w227:T24[])
                        n173 = for {
                          tunnel: w227 -> [w231] mode=indexing
                          n174 = Unbundle By Name(w231) -> ("GPIB Address"=w230:string)
                          n175 = call "Set_BSA_Coincidence.vi"("GPIB address"=w230, "Set Coincidence"=enum16{"Slave", "Master", "Private"}."Master") -> ()  [unwired: 1 in, 5 out]
                        }
                      }
                    }
                  }
                }
              }
              frame "BSA F60" {
                n176 = disable-structure shown="TARGET_TYPE==Windows" {
                  disable-tunnel: w233 -> [_ w234]
                  frame condition #0 (active) {
                  }
                  frame condition #1 {
                    n177 = while {
                      tunnel: w234 -> [w237]
                      stop <- w235 continue-if-true
                      n178 = call "Edit_BSA_IP.vi"("Show Panel"=w237) -> ("Run LDA Diagnostic Out"=w236:bool)  [unwired: 2 out]
                      n179 = case shown="False" w236 {
                        tunnel: [FALSE w239] -> w235
                        frame False {
                        }
                        frame True {
                          n180 = call "F60_Diagnostic.vi"() -> ("Edit BSA Setup Out"=w239:bool)  [unwired: 11 in]
                        }
                      }
                    }
                  }
                }
              }
            }
          }
        }
      }
      frame #9 {
        w248 = Save_Data."Save No Data" ("File")
        w264 = Post_Process."Take New Data"  # Post Process
        n181 = global read "Trav_pos_global.vi" "Meas Setup Number"() -> (w244:i32)
        n182 = Not Equal?(x=Setup."Run Program" ("setup"), y=w263) -> (x != y?=w249:bool)
        n183 = call "Current_Filepath.vi"("Filename in"="Results file", "Data Type"="Results") -> ("Filename Out"=w242:path)
        n184 = global read "Meas_global.vi" "Remote control"() -> (w260:bool)
        n185 = global read "Meas_global.vi" "Post Process"() -> (w251:T5)
        n186 = Equal?(x="File", y=w248) -> (x = y?=w258:bool)
        n187 = case shown="1, Default" w244 {
          tunnel: [w267 w269] -> w245
          tunnel: w242 -> [w267 w276]
          tunnel: w244 -> [_ w277]
          frame 0 {
          }
          frame 1, Default {
            n188 = Add(x=96, y=w277) -> (x+y=w279:i32)
            n189 = Build Array(w279) -> (w280:i32[])
            n190 = Strip Path(path=w276) -> (stripped path=w270:path, name=w275:string)
            n191 = Byte Array To String(unsigned byte array=w280) -> (string=w273:string)
            n192 = call "Add_filename_suffix.vi"("Filename"=w275) -> ("Original Suffix"=w272:string, "Base name"=w274:string)  [unwired: 1 in, 2 out]
            n193 = Format Into String(format string="%s_%s%s", w274, w273, w272) -> (resulting string=w271:string)  [unwired: 2 in, 1 out]
            n194 = Build Path(base path=w270, name or relative path=w271) -> (appended path=w269:path)
          }
        }
        n195 = Equal?(x=w251, y=w264) -> (x = y?=w250:bool)
        n196 = And(x=w260, y=w250) -> (x .and. y?=w256:bool)
        n197 = Compound Arithmetic op=AND(w258, invert w260, w250, invert w249) -> (w259:bool)
        n198 = while {
          shift-left: _ -> [w285]
          shift-right: [w282] -> _
          tunnel: "File" -> [w283]
          tunnel: [w286] -> w257
          tunnel: w259 -> [w282]
          stop <- FALSE continue-if-true
          n199 = Compound Arithmetic op=AND(w282, invert w285) -> (w284:bool)
          n200 = case shown="True" w284 {
            tunnel: [w287 w290] -> w286
            tunnel: w283 -> [w287 _]
            frame False {
            }
            frame True {
              n201 = Two Button Dialog(message="Do you wish to save the data?", 1:"Save Data" ("F button name (\"Cancel\")"), 2:"Save No Data" ("T button name (\"OK\")")) -> (T button?=w291:bool)
              n202 = Select(t=Save_Data."Save No Data" ("File"), s=w291, f=Save_Data."Save Data" ("File")) -> (s? t:f=w290:T9)
            }
          }
        }
        n203 = Equal?(x=w248, y=w257) -> (x = y?=w247:bool)
        n204 = Or(x=w247, y=w249) -> (x .or. y?=w262:bool)
        n205 = case shown="False" w262 {
          tunnel: w245 -> [w307 w315]
          tunnel: [w306 w315] -> w265
          tunnel: "Raw data file" -> [w305 w316]
          tunnel: [w300 w316] -> w254
          tunnel: w263 -> [w304 _]
          tunnel: w257 -> [w303 _]
          tunnel: [w301 T12."Save no data" ("File output")] -> w252
          tunnel: [w302 w313] -> w246
          tunnel: w256 -> [_ w310]
          tunnel: w249 -> [_ w309]
          tunnel: w243 -> [w299 _]
          frame False {
            n206 = call "File_setup.vi"("Measurement is top level?"=w299, "Results file"=w307, "Raw data file"=w305, "setup"=w304, "File"=w303) -> ("Results file output"=w306:path, "Raw data file output"=w300:path, "Raw data option"=w302:enum16{"Save raw data", "Raw data not saved"}, "File output"=w301:T12)
          }
          frame True {
            w311 = enum16{"Save raw data", "Raw data not saved"}."Raw data not saved"  # Raw data option
            n207 = global read "Meas_global.vi" "Raw data option"() -> (w312:enum16{"Save raw data", "Raw data not saved"})
            n208 = Compound Arithmetic op=AND(w310, invert w309) -> (w308:bool)
            n209 = Select(t=w312, s=w308, f=w311) -> (s? t:f=w313:enum16{"Save raw data", "Raw data not saved"})
          }
        }
        n210 = case shown="\"Save raw data\"" w246 {
          tunnel: w254 -> [w296 w298]
          tunnel: [w296 w297] -> w253
          frame "Raw data not saved" {
          }
          frame "Save raw data" {
            n211 = call "Find_Unique_Filename.vi"("Path In"=w298) -> ("Unique Path Out"=w297:path)  [unwired: 1 in, 1 out]
          }
        }
        n212 = case shown="\"Save data in new files\", Default" w252 {
          tunnel: w265 -> [_ w295]
          frame "Save no data" {
          }
          frame "Save data in new files", Default {
            n213 = local write "Results file"(w295) -> ()
            n214 = global write "Meas_global.vi" "Results file"(w295) -> ()
          }
        }
        n215 = global write "Meas_global.vi" "Raw data option"(w246) -> ()
        n216 = global write "Meas_global.vi" "File"(w252) -> ()
        n217 = global write "Meas_global.vi" "Raw data file"(w253) -> ()
        n218 = local write "Raw data file"(w253) -> ()
        n219 = local write "File"(w257) -> ()
      }
      frame #10 {
        n220 = global read "Meas_global.vi" "Ch & spans"() -> (w317:T25[])
        n221 = local read "Block average display control"() -> (w322:cluster{"Name":string, "Include":bool}[])
        n222 = global read "Meas_global.vi" "Velocity Cluster Array"() -> (w321:T26[])
        n223 = global write "Meas_global.vi" "Ch & spans + mod limits"(w317) -> ()
        n224 = global read "Meas_global.vi" "Analysis Info cluster"() -> (w327:T19[])
        n225 = call "Determine_Meas_Analysis.vi"("Analogue Channels"=w327) -> ("Analysis Info Cluster"=w324:T19[], "Analysis Type Array"=w326:T27[])
        n226 = for {
          tunnel: w324 -> [w337] mode=indexing
          tunnel: w322 -> [w336]
          tunnel: w321 -> [w334]
          tunnel: [w328] -> w320 mode=indexing
          tunnel: [w331] -> w319 mode=indexing
          tunnel: [w330] -> w318 mode=indexing
          i -> [w335]
          w329 = nan ("Mean % Err")
          n227 = Unbundle By Name(w337) -> ("Inst name"=w328:string)
          n228 = Index Array(array=w334, index=w335) -> (element=w333:T26)
          n229 = Index Array(array=w336, index=w335) -> (element=w332:cluster{"Name":string, "Include":bool})
          n230 = Bundle By Name(cluster=w332, "Name"=w328) -> (w331:cluster{"Name":string, "Include":bool})
          n231 = Bundle By Name(cluster=w333, "Name"=w328, "Mean % Err"=w329, "% u'/U"=w329) -> (w330:T26)
        }
        n232 = Build Array (concatenate)("Nothing", w320) -> (w323:string[])
        n233 = local write "Block average display control"(w319) -> ()
        n234 = global write "Meas_global.vi" "Analysis type array"(w326) -> ()
        n235 = global write "Meas_global.vi" "Analysis Info cluster"(w324) -> ()
        n236 = global write "Meas_global.vi" "Velocity Cluster Array"(w318) -> ()
        n237 = property on="Plot 1" class="Ring (strict)"("Strings []"=w323) -> ()  [unwired: 2 in, 2 out]
        n238 = property on="Plot 1" class="Ring (strict)"("Strings []"=w323) -> ()  [unwired: 2 in, 2 out]
        n239 = property on="Plot 2" class="Ring (strict)"("Strings []"=w323) -> ()  [unwired: 2 in, 2 out]
        n240 = property on="Plot 2" class="Ring (strict)"("Strings []"=w323) -> ()  [unwired: 2 in, 2 out]
      }
      frame #11 {
        n241 = global read "Meas_global.vi" "Analysis Info cluster"() -> (w350:T19[])
        n242 = for {
          tunnel: w350 -> [w354] mode=indexing
          tunnel: [w353] -> w349 mode=indexing
          tunnel: [w352] -> w340
          i -> [w352]
          n243 = Unbundle By Name(w354) -> ("Inst name"=w353:string)
        }
        n244 = Greater Than 0?(x=w340) -> (x > 0?=w339:bool)
        n245 = Select(t="Correlate?", s=w339, f=T6."Cross correlation off" ("Correlate?")) -> (s? t:f=w341:T6)
        n246 = case shown="\"Correlate without activating panel\"" w341 {
          tunnel: w349 -> [_ w359 w361]
          tunnel: [w356 w358 w360] -> w338
          frame "Cross correlation off" {
            n247 = Initialize Array(0) -> (w356:i32[][])  [unwired: 2 out]
          }
          frame "Show correlation panel" {
            w357 = FALSE  # OK
            n248 = call "Correlation_Display.vi"("Inst names"=w359, "OK"=w357) -> ("correlation array"=w358:i32[][])  [unwired: 2 in, 2 out]
          }
          frame "Correlate without activating panel" {
            n249 = call "Correlation_Display.vi"("Inst names"=w361, "OK"=TRUE) -> ("correlation array"=w360:i32[][])  [unwired: 2 in, 2 out]
          }
        }
        n250 = global read "Meas_global.vi" "Position"() -> (w348:T7)
        n251 = local write "Position"(w348) -> ()
        n252 = global write "Meas_global.vi" "correlate"(w338) -> ()
        n253 = Array Size(array=w338) -> (size(s)=w347:i32[])
        n254 = Index Array(array=w347, index=0) -> (element=w345:i32)
        n255 = Equal To 0?(x=w345) -> (x = 0?=w344:bool)
        n256 = case shown="True" w344 {
          frame False {
          }
          frame True {
            n257 = local write "Correlate?"(T6."Cross correlation off" ("Correlate?")) -> ()
          }
        }
      }
      frame #12 {
        n258 = stacked-sequence {
          seq-local: [w369 _] -> [_ w391]
          tunnel: w363 -> [w368 _]
          frame #0 {
            n259 = call "LDA+_An_Analysis_mode.vi"("Second Graph"="Second Graph", "First Graph"="First Graph") -> ("Second Graph out"=w364:T3, "First Graph out"=w366:T3)  [unwired: 6 out]
            n260 = case shown="False" w368 {
              tunnel: [w379 w390] -> w367
              tunnel: w366 -> [w378 w390]
              tunnel: [w377 w389] -> w365
              tunnel: w364 -> [w376 w389]
              frame False {
                w374 = Graph_Type."Show no graph" ("Plot Type")
                n261 = Unbundle By Name(w378) -> ("Save graph"=w380:u16)
                n262 = Unbundle By Name(w376) -> ("Save graph"=w375:u16)
                n263 = case shown="0, Default" w380 {
                  tunnel: [w386 w388] -> w379
                  tunnel: w378 -> [w387 w388]
                  tunnel: w374 -> [w385 _]
                  frame 0, Default {
                    n264 = Bundle By Name(cluster=w387, "Plot Type"=w385) -> (w386:T3)
                  }
                  frame 1 {
                  }
                }
                n265 = case shown="0, Default" w375 {
                  tunnel: [w382 w384] -> w377
                  tunnel: w376 -> [w383 w384]
                  tunnel: w374 -> [w381 _]
                  frame 0, Default {
                    n266 = Bundle By Name(cluster=w383, "Plot Type"=w381) -> (w382:T3)
                  }
                  frame 1 {
                  }
                }
              }
              frame True {
              }
            }
            n267 = local write "Second Graph"(w365) -> ()
            n268 = local write "First Graph"(w367) -> ()
            n269 = global write "Meas_global.vi" "Second Graph"(w365) -> ()
            n270 = global write "Meas_global.vi" "First Graph"(w367) -> ()
            n271 = Unbundle By Name(w365) -> ("Plot Type"=w373:T2)
            n272 = Unbundle By Name(w367) -> ("Plot Type"=w372:T2)
            n273 = Build Array(w372, w373) -> (w369:T2[])
          }
          frame #1 {
            n274 = global read "Meas_global.vi" "Insts for plotting"() -> (w392:u16[][])
            n275 = for {
              tunnel: w392 -> [w394] mode=indexing
              tunnel: w391 -> [w393] mode=indexing
              i -> [w395]
              n276 = stacked-sequence {
                seq-local: [w398 _] -> [_ w408]
                seq-local: [w399 _] -> [_ w407]
                tunnel: w395 -> [_ w411]
                tunnel: w394 -> [w397 _]
                tunnel: w393 -> [_ w403]
                frame #0 {
                  n277 = property on="Plot 1" class="Ring (strict)"() -> ("Strings []"=w396:string[])  [unwired: 2 in, 2 out]
                  n278 = Array To Cluster(array=w397) -> (cluster=w402:T29)
                  n279 = Unbundle(w402) -> ("Insts for plotting[0]"=w401:u16, "Insts for plotting[1]"=w400:u16)
                  n280 = Index Array(array=w396, index=w401) -> (element=w398:string)
                  n281 = Index Array(array=w396, index=w400) -> (element=w399:string)
                }
                frame #1 {
                  n282 = case shown="\"Auto-Corr\"" w403 {
                    tunnel: [u8 0 u8 0 u8 0 u8 0 u8 0 u8 1 u8 0] -> w415
                    tunnel: [u8 0 u8 0 u8 0 u8 0 u8 1 u8 1 u8 0] -> w414
                    tunnel: [u8 0 u8 0 u8 0 u8 0 u8 1 u8 1 u8 0] -> w413
                    tunnel: [u8 0 u8 0 u8 0 u8 0 u8 1 u8 0 u8 0] -> w412
                    tunnel: [FALSE TRUE TRUE TRUE TRUE TRUE TRUE] -> w406
                    tunnel: [u8 0 u8 0 u8 0 u8 2 u8 0 u8 0 u8 2] -> w405
                    tunnel: [u8 0 u8 4 u8 1 u8 2 u8 0 u8 0 u8 1] -> w404
                    frame "Show no graph" {
                    }
                    frame "Voltage trace" {
                    }
                    frame "Velocity trace" {
                    }
                    frame "Vel histogram" {
                    }
                    frame "Spectrum" {
                    }
                    frame "f.E(f) v Log f" {
                    }
                    frame "Auto-Corr" {
                    }
                  }
                  n283 = case shown="0, Default" w411 {
                    tunnel: w406 -> [w426 w437]
                    tunnel: w415 -> [w425 w436]
                    tunnel: w414 -> [w424 w435]
                    tunnel: w413 -> [w423 w434]
                    tunnel: w412 -> [w422 w433]
                    tunnel: u32 0 -> [w421 w432]
                    tunnel: u32 1 -> [w420 w430]
                    tunnel: w408 -> [w419 w431]
                    tunnel: w407 -> [w418 w429]
                    tunnel: w405 -> [w417 w428]
                    tunnel: w404 -> [w416 w427]
                    frame 0, Default {
                      n284 = property on="First plot" class="WFGraph (strict)"("Visible"=w426, "X Scale.Format & Precision:Format"=w425, "X Scale.Mapping Mode"=w424, "Y Scale.Format & Precision:Format"=w423, "Y Scale.Mapping Mode"=w422, "Active Plot"=w421, "Plot.Plot Name"=w419, "Active Plot"=w420, "Plot.Plot Name"=w418, "X Scale.Format & Precision:Precision"=w417, "Y Scale.Format & Precision:Precision"=w416) -> ()  [unwired: 2 in, 2 out]
                    }
                    frame 1 {
                      n285 = property on="2nd plot" class="WFGraph (strict)"("Visible"=w437, "X Scale.Format & Precision:Format"=w436, "X Scale.Mapping Mode"=w435, "Y Scale.Format & Precision:Format"=w434, "Y Scale.Mapping Mode"=w433, "Active Plot"=w432, "Plot.Plot Name"=w431, "Active Plot"=w430, "Plot.Plot Name"=w429, "X Scale.Format & Precision:Precision"=w428, "Y Scale.Format & Precision:Precision"=w427) -> ()  [unwired: 2 in, 2 out]
                    }
                  }
                }
              }
            }
          }
        }
      }
      frame #13 {
        n286 = local read "Second Graph"() -> (w498:T3)
        n287 = local read "First Graph"() -> (w497:T3)
        n288 = Unbundle By Name(w497) -> ("Plot 1"=w490:u16, "Plot 2"=w491:u16)
        n289 = Unbundle By Name(w498) -> ("Plot 1"=w492:u16, "Plot 2"=w493:u16)
        n290 = Build Array(w490, w491) -> (w494:u16[])
        n291 = Build Array(w492, w493) -> (w495:u16[])
        n292 = global read "Meas_global.vi" "Analysis Info cluster"() -> (w499:T19[])
        n293 = Decrement(x=w494) -> (x-1=w488:u16[])
        n294 = Decrement(x=w495) -> (x-1=w496:u16[])
        n295 = for {
          tunnel: w499 -> [w507]
          tunnel: w488 -> [w506] mode=indexing
          shift-right: [w500] -> _
          shift-left: u32 0 -> [w502]
          i -> [w501]
          n296 = Index Array(array=w507, index=w506) -> (element=w508:T19)
          n297 = Unbundle By Name(w508) -> ("Colour"=w503:u32)
          n298 = Equal?(x=w503, y=w502) -> (x = y?=w505:bool)
          n299 = Select(t=u32 13434624, s=w505, f=w503) -> (s? t:f=w500:u32)
          n300 = property on="First plot" class="WFGraph (strict)"("Active Plot"=w501, "Plot.Plot Color"=w500, "Plot.Fill/Point Color"=w500) -> ()  [unwired: 2 in, 2 out]
        }
        n301 = for {
          tunnel: w499 -> [w516]
          tunnel: w496 -> [w515] mode=indexing
          shift-right: [w511] -> _
          shift-left: u32 0 -> [w509]
          i -> [w514]
          n302 = Index Array(array=w516, index=w515) -> (element=w517:T19)
          n303 = Unbundle By Name(w517) -> ("Colour"=w510:u32)
          n304 = Equal?(x=w510, y=w509) -> (x = y?=w513:bool)
          n305 = Select(t=u32 13434624, s=w513, f=w510) -> (s? t:f=w511:u32)
          n306 = property on="2nd plot" class="WFGraph (strict)"("Active Plot"=w514, "Plot.Plot Color"=w511, "Plot.Fill/Point Color"=w511) -> ()  [unwired: 2 in, 2 out]
        }
      }
      frame #14 {
        n307 = global read "Meas_global.vi" "Remote control"() -> (w526:bool)
        n308 = global read "Meas_global.vi" "Post Process"() -> (w529:T5)
        n309 = global read "Meas_global.vi" "PWA Data"() -> (w518:T30)
        n310 = case shown="\"One Ch PWA\"" w518 {
          tunnel: [w530 w535] -> w520
          frame "No PWA Data" {
            n311 = local read "Desired Sampling freq (Hz)"() -> (w532:dbl)
            n312 = local read "No of samples"() -> (w531:i32)
            n313 = Divide(x=w531, y=w532) -> (x/y=w530:dbl)
          }
          frame "One Ch PWA" {
            n314 = local read "No of samples"() -> (w533:i32)
            n315 = global read "PWAtasksGLOBAL.vi" "PWA Freq. (Hz)"() -> (w534:dbl)
            n316 = global write "PWAtasksGLOBAL.vi" "PWA No. of Samples"(w533) -> ()
            n317 = Divide(x=w533, y=w534) -> (x/y=w535:dbl)
          }
        }
        n318 = global read "Meas_global.vi" "Averaging time (min)"() -> (w524:dbl)
        n319 = Equal?(x=Setup."Run Program" ("setup"), y=w523) -> (x = y?=w521:bool)
        n320 = Equal?(x=Post_Process."Take New Data" ("Post Process"), y=w529) -> (x = y?=w525:bool)
        n321 = Compound Arithmetic op=AND(w525, invert w519, invert w526, w521) -> (w527:bool)
        n322 = case shown="True" w527 {
          tunnel: w524 -> [_ w542]
          tunnel: w520 -> [_ w541]
          tunnel: w518 -> [_ w536]
          frame False {
          }
          frame True {
            n323 = global read "Meas_global.vi" "Board type"() -> (w539:T13)
            n324 = Equal?(x=w539, y=Board_Types."Server Channels" ("Board type")) -> (x = y?=w538:bool)
            n325 = case shown="False" w538 {
              tunnel: w542 -> [w552 _]
              tunnel: w541 -> [w545 _]
              tunnel: [w544 1 ("No of Blocks")] -> w537
              tunnel: w536 -> [w543 _]
              frame False {
                n326 = Multiply(x=w552, y=60.0) -> (x*y=w550:dbl)
                n327 = global read "Meas_global.vi" "LDA data"() -> (w554:enum16{"No LDA data", "Take LDA data"})
                n328 = Equal?(x=enum16{"No LDA data", "Take LDA data"}."Take LDA data" ("LDA data"), y=w554) -> (x = y?=w548:bool)
                n329 = Divide(x=w550, y=w545) -> (x/y=w549:dbl)
                n330 = Round Toward +Infinity(x=w549) -> (ceil(x): smallest int >= x=w547:dbl)
                n331 = To Long Integer(number=w547) -> (32bit integer=w546:i32)
                n332 = case shown="\"No PWA Data\"" w543 {
                  tunnel: w548 -> [w558 _]
                  tunnel: w546 -> [w556 w559]
                  tunnel: [w555 w559] -> w544
                  frame "No PWA Data" {
                    n333 = Select(t=99999 ("No of Blocks"), s=w558, f=w556) -> (s? t:f=w555:i32)
                  }
                  frame "One Ch PWA" {
                  }
                }
              }
              frame True {
              }
            }
            n334 = global write "Meas_global.vi" "Requested No of blocks"(w537) -> ()
            n335 = local write "No of Blocks"(w537) -> ()
          }
        }
      }
      frame #15 {
        n336 = case shown="\"Run Program\"" w561 {
          frame "Run Program" {
            n337 = call "Read_calibration_files.vi"() -> ()  [unwired: 1 out]
            n338 = global write "Meas_global.vi" "Repeat Measurement?"(FALSE ("Repeat Measurement?")) -> ()
          }
          frame "Show Setup", Default {
          }
        }
      }
      frame #16 {
        n339 = global read "Meas_global.vi" "Raw data option"() -> (w566:enum16{"Save raw data", "Raw data not saved"})
        n340 = Get Date/Time In Seconds() -> (seconds since 1Jan1904=w567:timestamp)
        n341 = To Double Precision Float(number=w567) -> (double precision float=w564:dbl)
        n342 = global read "Meas_global.vi" "Post Process"() -> (w565:T5)
        n343 = global read "Constants_global.vi" "Meas setups folder"() -> (w568:path)
        n344 = case shown="\"Run Program\"" w569 {
          tunnel: w568 -> [w572 w587 w610 w620]
          tunnel: w566 -> [w573 _ _ _]
          tunnel: w565 -> [w571 _ w609 w619]
          frame "Run Program" {
            n345 = case shown="\"Take New Data\"" w571 {
              tunnel: w573 -> [w575 _]
              tunnel: w572 -> [w574 _]
              frame "Take New Data" {
                n346 = case shown="\"Raw data not saved\"" w575 {
                  tunnel: w574 -> [_ w576]
                  frame "Save raw data" {
                  }
                  frame "Raw data not saved" {
                    w582 = FALSE  # Lock File
                    w578 = FALSE  # advisory dialog? (display:T)
                    w577 = FALSE  # append to file? (new file:F)
                    n347 = global read "Meas_global.vi" "Remote control"() -> (w579:bool)
                    n348 = call "Create_setup_string.vi"() -> ("Setup String"=w584:string)  [unwired: 1 out]
                    n349 = case shown="False" w579 {
                      tunnel: ["Current_Setup.xls" ("Setup filename") w586] -> w581
                      frame False {
                      }
                      frame True {
                        n350 = local read "Setup filename"() -> (w586:string)
                      }
                    }
                    n351 = call "Add_length_to_string.vi"("String in"=w584) -> ("String out"=w580:string)
                    n352 = Build Path(base path=w576, name or relative path=w581) -> (appended path=w583:path)
                    n353 = call "Write_Characters_To_File.vi"("file path (dialog if empty)"=w583, "advisory dialog? (display:T)"=w578, "character string"=w580, "append to file? (new file:F)"=w577, "Lock File"=w582) -> ()  [unwired: 4 out]
                  }
                }
              }
              frame "Post Process Raw Data File" {
              }
            }
          }
          frame "Save Current Setup" {
            n354 = stacked-sequence {
              seq-local: [w589 _ _] -> [_ w593 w599]
              seq-local: [w588 _ _] -> [_ w592 w598]
              tunnel: w587 -> [w591 _ _]
              frame #0 {
                w590 = FALSE  # Save New File?
                n355 = call "Save_current_setup.vi"("Save New File?"=w590, "Folder"=w591) -> ("Cancelled?"=w588:bool, "Saved filepath"=w589:path)  [unwired: 2 out]
              }
              frame #1 {
                n356 = case shown="False" w592 {
                  tunnel: w593 -> [w594 _]
                  frame False {
                    n357 = global read "Meas_global.vi" "New Setup String"() -> (w597:string)
                    n358 = call "Input_Instrument_Positions.vi"("Filepath to Save"=w594) -> ("Output string"=w596:string)  [unwired: 1 out]
                    n359 = Concatenate Strings(w597, w596) -> (w595:string)
                    n360 = global write "Meas_global.vi" "New Setup String"(w595) -> ()
                  }
                  frame True {
                  }
                }
              }
              frame #2 {
                n361 = case shown="False" w598 {
                  tunnel: w599 -> [w604 _]
                  frame False {
                    w606 = FALSE  # append to file? (new file:F)
                    w607 = FALSE  # advisory dialog? (display:T)
                    w608 = FALSE  # Lock File
                    n362 = call "Create_setup_string.vi"() -> ("Setup String"=w602:string)  [unwired: 1 out]
                    n363 = call "Replace_data_in_setup_string.vi"("New data string"="", "Input string"=w602, "Variable name"="Comments") -> ("Appended string"=w600:string)
                    n364 = call "Add_length_to_string.vi"("String in"=w600) -> ("String out"=w605:string)
                    n365 = call "Write_Characters_To_File.vi"("file path (dialog if empty)"=w604, "advisory dialog? (display:T)"=w607, "character string"=w605, "append to file? (new file:F)"=w606, "Lock File"=w608) -> ()  [unwired: 4 out]
                  }
                  frame True {
                  }
                }
              }
            }
          }
          frame "Show Setup" {
            n366 = case shown="\"Take New Data\"" w609 {
              tunnel: w610 -> [w618 _]
              frame "Take New Data" {
                w613 = FALSE  # append to file? (new file:F)
                w614 = FALSE  # advisory dialog? (display:T)
                w615 = FALSE  # Lock File
                n367 = call "Create_setup_string.vi"() -> ("Setup String"=w616:string)  [unwired: 1 out]
                n368 = Build Path(base path=w618, name or relative path="Current_Setup.xls" ("Setup filename")) -> (appended path=w612:path)
                n369 = call "Add_length_to_string.vi"("String in"=w616) -> ("String out"=w611:string)
                n370 = call "Write_Characters_To_File.vi"("file path (dialog if empty)"=w612, "advisory dialog? (display:T)"=w614, "character string"=w611, "append to file? (new file:F)"=w613, "Lock File"=w615) -> ()  [unwired: 4 out]
              }
              frame "Post Process Raw Data File" {
              }
            }
          }
          frame "Setup Front Panel" {
            n371 = case shown="\"Take New Data\"" w619 {
              tunnel: w620 -> [w621 _]
              frame "Take New Data" {
                w624 = FALSE  # append to file? (new file:F)
                w625 = FALSE  # advisory dialog? (display:T)
                w626 = FALSE  # Lock File
                n372 = call "Create_setup_string.vi"() -> ("Setup String"=w627:string)  [unwired: 1 out]
                n373 = Build Path(base path=w621, name or relative path="Current_Setup.xls" ("Setup filename")) -> (appended path=w623:path)
                n374 = call "Add_length_to_string.vi"("String in"=w627) -> ("String out"=w622:string)
                n375 = call "Write_Characters_To_File.vi"("file path (dialog if empty)"=w623, "advisory dialog? (display:T)"=w625, "character string"=w622, "append to file? (new file:F)"=w624, "Lock File"=w626) -> ()  [unwired: 4 out]
              }
              frame "Post Process Raw Data File" {
              }
            }
          }
        }
        n376 = call "Program_Active.vi"() -> ()  [unwired: 1 in]
        n377 = global write "Meas_global.vi" "Actual Measurement time (min)"(0.0 ("Max Measurement time (min)")) -> ()
        n378 = global write "Meas_global.vi" "Current Block No"(0 ("Current Block No")) -> ()
      }
      frame #17 {
        n379 = case shown="\"Run Program\"" w632 {
          tunnel: w629 -> [w634 _]
          tunnel: w631 -> [_ w821]
          tunnel: w630 -> [w633 _]
          frame "Run Program" {
            # "PWA"
            # "LDA"
            # "An"
            n380 = stacked-sequence {
              seq-local: [w642 _] -> [_ w664]
              seq-local: [w641 _] -> [_ w663]
              seq-local: [w640 _] -> [_ w662]
              seq-local: [w638 _] -> [_ w661]
              seq-local: [w636 _] -> [_ w658]
              seq-local: [w635 _] -> [_ w657]
              tunnel: w634 -> [_ w660]
              tunnel: w633 -> [_ w659]
              frame #0 {
                n381 = global read "Trav_pos_global.vi" "Dummy Measurement?"() -> (w637:bool)
                n382 = case shown="False" w637 {
                  tunnel: [w649 u16[][] [] ("LDA Binary output")] -> w642
                  tunnel: [w648 w651] -> w641
                  tunnel: [w647 dbl[][] [] ("Voltage output")] -> w640
                  tunnel: [w646 TRUE ("EOF?")] -> w639
                  tunnel: [w645 T14 {"Started"=0.0, "Ended"=0.0, "Analogue Frequency Hz"=1000.0} ("Block Timings")] -> w638
                  tunnel: [w644 w651] -> w636
                  tunnel: [w643 ""] -> w635
                  frame False {
                    n383 = call "Get_data.vi"() -> ("EOF? and Error status"=w646:bool, "Voltage output"=w647:dbl[][], "Analogue Binary"=w648:i16[][], "LDA Binary output"=w649:u16[][], "Block Timings"=w645:T14, "PWA Binary"=w644:i16[][], "Block Header"=w643:string)  [unwired: 5 out]
                  }
                  frame True {
                    w651 = i16[][] [] ("Analogue Binary")
                  }
                }
                n384 = case shown="True" w639 {
                  frame False {
                  }
                  frame True {
                    n385 = local write "No of Blocks"(1 ("No of Blocks")) -> ()
                  }
                }
              }
              frame #1 {
                n386 = while {
                  tunnel: w660 -> [w670]
                  shift-left: w661 -> [w671]
                  shift-right: [w672] -> _
                  shift-left: w662 -> [w676]
                  shift-right: [w679] -> _
                  shift-left: w663 -> [w677]
                  shift-right: [w680] -> _
                  shift-left: w664 -> [w678]
                  shift-right: [w681] -> _
                  tunnel: w659 -> [w669]
                  shift-right: [w668] -> _
                  shift-left: w658 -> [w667]
                  shift-right: [w666] -> _
                  shift-left: w657 -> [w665]
                  i -> [w673]
                  stop <- w682 continue-if-true
                  n387 = Increment(x=w673) -> (x+1=w683:i32)
                  n388 = stacked-sequence {
                    seq-local: [_ _ _ _ _ "Block average display control" _ _ _ _] -> [_ _ _ _ _ _ w778 _ _ _]
                    seq-local: [_ _ _ _ _ _ w775 _ _ _] -> [_ _ _ _ _ _ _ w789 _ _]
                    seq-local: [w719 _ _ _ _ _ _ _ _ _] -> [_ w725 _ _ w761 _ _ _ _ w819]
                    seq-local: [_ _ w730 _ _ _ _ _ _ _] -> [_ _ _ _ w759 _ _ _ _ _]
                    seq-local: [_ _ _ w751 _ _ _ _ _ _] -> [_ _ _ _ w760 _ _ _ _ _]
                    tunnel: w683 -> [w718 _ _ _ w763 w771 _ _ _ _]
                    tunnel: [_ _ _ _ _ _ _ _ _ w819] -> w682
                    tunnel: w673 -> [_ _ _ _ _ _ _ _ _ _]
                    tunnel: w678 -> [_ _ _ w749 _ _ _ _ _ _]
                    tunnel: w677 -> [_ _ _ w748 _ _ _ _ _ _]
                    tunnel: w676 -> [_ _ _ w755 _ _ _ _ _ _]
                    tunnel: "stop" -> [w721 _ _ _ _ _ _ _ _ _]
                    tunnel: "No of Blocks" -> [w720 _ _ _ _ _ _ _ _ _]
                    tunnel: w671 -> [_ _ _ w753 _ _ _ _ _ _]
                    tunnel: w670 -> [_ _ w729 w750 _ _ _ _ _ _]
                    tunnel: w669 -> [_ _ w731 _ _ _ _ _ _ _]
                    tunnel: w667 -> [_ _ _ w747 _ _ _ _ _ _]
                    tunnel: w665 -> [w717 _ _ _ _ _ _ _ _ _]
                    frame #0 {
                      n389 = global write "Plug_in_data_global.vi" "Block Header"(w717) -> ()
                      n390 = Less Or Equal?(x=w720, y=w718) -> (x <= y?=w723:bool)
                      n391 = Or(x=w721, y=w723) -> (x .or. y?=w722:bool)
                      n392 = global write "Meas_global.vi" "Current Block No"(w718) -> ()
                      n393 = Not(x=w722) -> (.not. x?=w719:bool)
                    }
                    frame #1 {
                      n394 = call "Program_Active.vi"() -> ()  [unwired: 1 in]
                      n395 = call "Text_without_format.vi"("Input string"="Comments") -> ("Output string"=w726:string)
                      n396 = global write "Meas_global.vi" "Position"("Position") -> ()
                      n397 = local write "Comments"(w726) -> ()
                      n398 = global write "Meas_global.vi" "Comments"(w726) -> ()
                      n399 = Not(x=w725) -> (.not. x?=w724:bool)
                      n400 = global write "Meas_global.vi" "Processing last block?"(w724) -> ()
                      n401 = global write "PWAtasksGLOBAL.vi" "STOP"(w724) -> ()
                    }
                    frame #2 {
                      n402 = case shown="False" w729 {
                        tunnel: w731 -> [w743 _]
                        tunnel: [w732 FALSE] -> w730
                        frame False {
                          w740 = 1.5  # To allow for overhead
                          n403 = Get Date/Time In Seconds() -> (seconds since 1Jan1904=w745:timestamp)
                          n404 = global read "Meas_global.vi" "Averaging time (min)"() -> (w739:dbl)
                          n405 = To Double Precision Float(number=w745) -> (double precision float=w744:dbl)
                          n406 = Subtract(x=w744, y=w743) -> (x-y=w742:dbl)
                          n407 = global read "Meas_global.vi" "LDA data"() -> (w736:enum16{"No LDA data", "Take LDA data"})
                          n408 = Divide(x=w742, y=60.0 ("To convert to minutes")) -> (x/y=w738:dbl)
                          n409 = Equal?(x=enum16{"No LDA data", "Take LDA data"}."Take LDA data" ("LDA data"), y=w736) -> (x = y?=w733:bool)
                          n410 = Multiply(x=w740, y=w739) -> (x*y=w737:dbl)
                          n411 = Greater?(x=w738, y=w737) -> (0:w734:bool)
                          n412 = And(x=w733, y=w734) -> (x .and. y?=w732:bool)
                        }
                        frame True {
                        }
                      }
                    }
                    frame #3 {
                      n413 = call "Process_data.vi"("PWA Binary"=w747, "Analogue Binary"=w748, "LDA Binary output"=w749, "Analogue volts"=w755, "Measurement top level?"=w750, "Block Timings"=w753) -> ("Vel stat display"=→"Statistics":string[][], "First Plot data"=→"First plot":cluster{"Xo":dbl, "Delta X":dbl, dbl[]}[], "Second Plot data"=→"2nd plot":cluster{"Xo":dbl, "Delta X":dbl, dbl[]}[], "Max Measurement time up"=w751:bool)
                    }
                    frame #4 {
                      n414 = global read "Meas_global.vi" "stop"() -> (w758:bool)
                      n415 = Compound Arithmetic op=OR(w758, w759, w760) -> (w757:bool)
                      n416 = And(x=w761, y=w757) -> (x .and. y?=w762:bool)
                      n417 = case shown="True" w762 {
                        tunnel: w763 -> [_ w764]
                        frame False {
                        }
                        frame True {
                          n418 = Increment(x=w764) -> (x+1=w765:i32)
                          n419 = local write "No of Blocks"(w765) -> ()
                        }
                      }
                    }
                    frame #5 {
                      n420 = global read "Meas_global.vi" "Actual Measurement time (min)"() -> (→"Measurement time (min)":dbl)
                      n421 = global read "Meas_global.vi" "Actual Sampling rate (Hz)"() -> (→"Actual Sampling freq":dbl)
                      n422 = call "Display_blocks.vi"("Block No"=w771, "Block average display"="Block average display control") -> ("u^4"=→"u^4":dbl[][], "u^3"=→"u^3":dbl[][], "uv"=→"uv":dbl[][], "u^2"=→"u^2" →"Array u^2":dbl[][], "U"=→"U" →"Array U":dbl[][])  [unwired: 4 out]
                    }
                    frame #6 {
                      n423 = global read "Meas_global.vi" "Analysis Info cluster"() -> (w777:T19[])
                      n424 = for {
                        tunnel: w778 -> [w783] mode=indexing
                        shift-right: [w779] -> w775
                        shift-left: u32[] [] -> [w780]
                        tunnel: w777 -> [w782] mode=indexing
                        n425 = Unbundle By Name(w783) -> ("Include"=w781:bool)
                        n426 = case shown="True" w781 {
                          tunnel: w782 -> [_ w788]
                          tunnel: w780 -> [w784 w786]
                          tunnel: [w784 w785] -> w779
                          frame False {
                          }
                          frame True {
                            n427 = Unbundle By Name(w788) -> ("Colour"=w787:u32)
                            n428 = Build Array (concatenate)(w786, w787) -> (w785:u32[])
                          }
                        }
                      }
                    }
                    frame #7 {
                      n429 = for {
                        tunnel: w789 -> [w790] mode=indexing
                        i -> [w791]
                        n430 = property on="U" class="WFGraph (strict)"("Active Plot"=w791, "Plot.Plot Color"=w790, "Plot.Fill/Point Color"=w790) -> ()  [unwired: 2 in, 2 out]
                        n431 = property on="u^3" class="WFGraph (strict)"("Active Plot"=w791, "Plot.Plot Color"=w790, "Plot.Fill/Point Color"=w790) -> ()  [unwired: 2 in, 2 out]
                        n432 = property on="u^4" class="WFGraph (strict)"("Active Plot"=w791, "Plot.Plot Color"=w790, "Plot.Fill/Point Color"=w790) -> ()  [unwired: 2 in, 2 out]
                        n433 = property on="u^2" class="WFGraph (strict)"("Active Plot"=w791, "Plot.Plot Color"=w790, "Plot.Fill/Point Color"=w790) -> ()  [unwired: 2 in, 2 out]
                      }
                    }
                    frame #8 {
                      n434 = case shown="True" "Pause" {
                        frame False {
                        }
                        frame True {
                          n435 = global read "Meas_global.vi" "Post Process"() -> (w793:T5)
                          n436 = case shown="\"Take New Data\"" w793 {
                            frame "Take New Data" {
                              n437 = call "Program_Active_Client.vi"("Mode"=enum16{"Program Active", "Traverse Level State"}."Program Active", "Time till next contact (Sec)"=12000.0, "Traverse level State"=Traverse_Level_State."Running") -> ()  [unwired: 3 out]
                              n438 = while {
                                i -> [w800]
                                stop <- w801 continue-if-true
                                n439 = Quotient & Remainder(x=w800, y=10) -> (x-y*floor(x/y)=w798:i32)  [unwired: 1 out]
                                n440 = Equal To 0?(x=w798) -> (x = 0?=w797:bool)
                                n441 = stacked-sequence {
                                seq-local: [_ w803 _ _] -> [_ _ w805 _]
                                tunnel: [_ w803 _ _] -> w801
                                tunnel: w797 -> [_ _ _ w807]
                                frame #0 {
                                "Pause message" <- "Measurement Program Paused!!!!" ("Pause message")
                                }
                                frame #1 {
                                n442 = global write "Trav_pos_global.vi" "Paused During Row?"(TRUE ("Paused During Row?")) -> ()
                                n443 = local read "Pause"() -> (w803:bool)
                                }
                                frame #2 {
                                n444 = property on="Pause message" class="Str"("Blinking"=w805, "Visible"=w805) -> ()  [unwired: 2 in, 2 out]
                                n445 = Wait Until Next ms Multiple(millisecond multiple=u32 1000) -> ()  [unwired: 1 out]
                                }
                                frame #3 {
                                n446 = case shown="False" w807 {
                                frame False {
                                }
                                frame True {
                                n447 = Current VI's Path() -> (path=w808:path)
                                n448 = call "Bring_to_front.vi"("path"=w808) -> ()
                                }
                                }
                                }
                                }
                              }
                            }
                            frame "Post Process Raw Data File" {
                              n449 = stacked-sequence {
                                seq-local: [_ w811 _ _] -> [_ _ _ w818]
                                frame #0 {
                                n450 = property on="PP next block" class="Bool (strict)"("Visible"=TRUE) -> ()  [unwired: 2 in, 2 out]
                                n451 = local write "PP next block"(FALSE ("PP next block")) -> ()
                                }
                                frame #1 {
                                n452 = while {
                                tunnel: [w815] -> w811
                                stop <- w812 stop-if-true
                                n453 = local read "stop"() -> (w815:bool)
                                n454 = local read "Pause"() -> (w813:bool)
                                n455 = Compound Arithmetic op=OR(w815, "PP next block", invert w813) -> (w812:bool)
                                n456 = case shown="False" w812 {
                                frame False {
                                n457 = Wait (ms)(milliseconds to wait=u32 200) -> ()  [unwired: 1 out]
                                }
                                frame True {
                                }
                                }
                                }
                                }
                                frame #2 {
                                n458 = property on="PP next block" class="Bool (strict)"("Visible"=FALSE) -> ()  [unwired: 2 in, 2 out]
                                }
                                frame #3 {
                                n459 = Stop(stop? (T)=w818) -> ()
                                }
                              }
                            }
                          }
                        }
                      }
                    }
                    frame #9 {
                      n460 = global read "Meas_global.vi" "Diagnostic info"() -> (→"BSA Diagnostic info":string[][])
                    }
                  }
                  n461 = stacked-sequence {
                    seq-local: [w685 _ _] -> [_ w695 _]
                    seq-local: [_ w694 _] -> [_ _ w715]
                    tunnel: [_ w698 _] -> w681
                    tunnel: [_ w697 _] -> w680
                    tunnel: [_ w696 _] -> w679
                    tunnel: "No of Blocks" -> [w690 _ _]
                    tunnel: "stop" -> [w688 _ _]
                    tunnel: w673 -> [w686 _ w714]
                    tunnel: [_ w693 _] -> w672
                    tunnel: [_ w692 _] -> w668
                    tunnel: [_ w691 _] -> w666
                    frame #0 {
                      n462 = Increment(x=w686) -> (x+1=w684:i32)
                      "Current Block No" <- w684
                      n463 = Less Or Equal?(x=w690, y=w684) -> (x <= y?=w689:bool)
                      n464 = Or(x=w689, y=w688) -> (x .or. y?=w687:bool)
                      n465 = Not(x=w687) -> (.not. x?=w685:bool)
                      n466 = global write "Meas_global.vi" "Current Block No"(w684) -> ()
                    }
                    frame #1 {
                      n467 = case shown="True" w695 {
                        tunnel: [u16[][] [] ("LDA Binary output") w711] -> w698
                        tunnel: [w700 w710] -> w697
                        tunnel: [dbl[][] [] ("Voltage output") w709] -> w696
                        tunnel: [FALSE ("EOF?") w708] -> w694
                        tunnel: [T14 {"Started"=0.0, "Ended"=0.0, "Analogue Frequency Hz"=200.0} ("Block Timings") w707] -> w693
                        tunnel: [w700 w706] -> w692
                        tunnel: ["" w705] -> w691
                        frame False {
                          w700 = i16[][] [] ("Analogue Binary")
                        }
                        frame True {
                          n468 = call "Get_data.vi"() -> ("EOF? and Error status"=w708:bool, "Voltage output"=w709:dbl[][], "Analogue Binary"=w710:i16[][], "LDA Binary output"=w711:u16[][], "Block Timings"=w707:T14, "PWA Binary"=w706:i16[][], "Block Header"=w705:string)  [unwired: 5 out]
                        }
                      }
                    }
                    frame #2 {
                      n469 = Increment(x=w714) -> (x+1=w712:i32)
                      n470 = Increment(x=w712) -> (x+1=w713:i32)
                      n471 = case shown="True" w715 {
                        tunnel: w713 -> [_ w716]
                        frame False {
                        }
                        frame True {
                          n472 = local write "No of Blocks"(w716) -> ()
                        }
                      }
                    }
                  }
                }
              }
            }
          }
          frame "Setup Front Panel", Default {
            n473 = stacked-sequence {
              seq-local: [w822 _ _ _ _ _ _] -> [_ _ _ _ _ w896 _]
              seq-local: [_ w828 _ _ _ _ _] -> [_ _ _ _ _ w895 _]
              seq-local: [_ _ _ w859 _ _ _] -> [_ _ _ _ _ w894 _]
              seq-local: [_ _ _ _ w872 _ _] -> [_ _ _ _ _ w892 _]
              seq-local: [_ w827 _ _ _ _ _] -> [_ _ _ _ _ _ w909]
              seq-local: [_ _ w853 _ _ _ _] -> [_ _ _ _ _ w891 _]
              tunnel: w821 -> [_ w829 _ _ _ _ _]
              frame #0 {
                n474 = Build Array("Name", "Channel", "High limit", "Low limit") -> (w822:string[])
              }
              frame #1 {
                n475 = global read "Meas_global.vi" "LDA data"() -> (w827:enum16{"No LDA data", "Take LDA data"})
                n476 = case shown="\"Take LDA data\"" w827 {
                  tunnel: w829 -> [_ w840]
                  tunnel: [string[][] [] w837] -> w828
                  frame "No LDA data" {
                  }
                  frame "Take LDA data" {
                    n477 = case shown="\"2D\"" w840 {
                      tunnel: [string[] [] w846] -> w838
                      frame "1D" {
                      }
                      frame "2D" {
                        n478 = global read "LDA_meas_global_2.vi" "Max Vel BSA2"() -> (w845:dbl)
                        n479 = global read "LDA_meas_global_2.vi" "Min Vel BSA2"() -> (w844:dbl)
                        n480 = global read "LDA_meas_global_2.vi" "Vel Comp BSA2"() -> (w847:string)
                        n481 = Format Into String(format string="%.1f m/s" ("Format String"), w844) -> (resulting string=w852:string)  [unwired: 2 in, 1 out]
                        n482 = Format Into String(format string="%.1f m/s" ("Format String"), w845) -> (resulting string=w851:string)  [unwired: 2 in, 1 out]
                        n483 = Build Array("LDA", w847, w851, w852) -> (w846:string[])
                      }
                    }
                    n484 = global read "LDA_meas_global_1.vi" "Max Vel BSA1"() -> (w832:dbl)
                    n485 = global read "LDA_meas_global_1.vi" "Vel Comp BSA1"() -> (w841:string)
                    n486 = global read "LDA_meas_global_1.vi" "Min Vel BSA1"() -> (w831:dbl)
                    n487 = Format Into String(format string="%.1f m/s" ("Format String"), w831) -> (resulting string=w833:string)  [unwired: 2 in, 1 out]
                    n488 = Format Into String(format string="%.1f m/s" ("Format String"), w832) -> (resulting string=w834:string)  [unwired: 2 in, 1 out]
                    n489 = Build Array("LDA", w841, w834, w833) -> (w839:string[])
                    n490 = Build Array(w839, w838) -> (w837:string[][])
                  }
                }
              }
              frame #2 {
                n491 = global read "Meas_global.vi" "PWA Data"() -> (w854:T30)
                n492 = case shown="\"One Ch PWA\"" w854 {
                  tunnel: [string[][] [] w856] -> w853
                  frame "No PWA Data" {
                  }
                  frame "One Ch PWA" {
                    n493 = Build Array("PWA") -> (w857:string[])
                    n494 = Build Array(w857) -> (w856:string[][])
                  }
                }
              }
              frame #3 {
                n495 = global read "Meas_global.vi" "Ch & spans"() -> (w860:T25[])
                n496 = for {
                  tunnel: w860 -> [w871] mode=indexing
                  tunnel: [w867] -> w859 mode=indexing
                  n497 = Unbundle By Name(w871) -> ("Var name"=w870:string, "Ch No"=w869:i16, "high limit (10V)"=w864:sgl, "low limit (-10V)"=w863:sgl)
                  n498 = Format Into String(format string="%.1f Volts" ("Format String"), w864) -> (resulting string=w862:string)  [unwired: 2 in, 1 out]
                  n499 = Format Into String(format string="%.1f Volts" ("Format String"), w863) -> (resulting string=w861:string)  [unwired: 2 in, 1 out]
                  n500 = Number To Decimal String(number=w869) -> (decimal integer string=w868:string)  [unwired: 1 out]
                  n501 = Build Array(w870, w868, w862, w861) -> (w867:string[])
                }
              }
              frame #4 {
                n502 = global read "Meas_global.vi" "Analysis Info cluster"() -> (w880:T19[])
                n503 = for {
                  tunnel: w880 -> [w890] mode=indexing
                  tunnel: [w889] -> w878 mode=indexing
                  n504 = Unbundle By Name(w890) -> ("Inst name"=w889:string)
                }
                n505 = global read "Meas_global.vi" "correlate"() -> (w879:i32[][])
                n506 = for {
                  tunnel: w879 -> [w885] mode=indexing
                  tunnel: w878 -> [w884]
                  tunnel: "Correlating" -> [w883]
                  tunnel: [w881] -> w873 mode=indexing
                  n507 = for {
                    tunnel: w885 -> [w888] mode=indexing
                    tunnel: w884 -> [w887]
                    tunnel: [w886] -> w882 mode=indexing
                    n508 = Index Array(array=w887, index=w888) -> (element=w886:string)
                  }
                  n509 = Build Array (concatenate)(w883, w882) -> (w881:string[])
                }
                n510 = Initialize Array("", 5 ("Dimension Size")) -> (w874:string[])
                n511 = Build Array (concatenate)(w874, w873) -> (w872:string[][])
              }
              frame #5 {
                n512 = Build Array (concatenate)(w896, w895, w891, w894, w892) -> (w893:string[][])
                n513 = local write "Statistics"(w893) -> ()
              }
              frame #6 {
                n514 = global read "Meas_global.vi" "Board type"() -> (w907:T13)
                n515 = global read "Meas_global.vi" "Continuous time trace?"() -> (w908:bool)
                n516 = Equal?(x=w907, y=Board_Types."ADC488" ("Board type")) -> (x = y?=w905:bool)
                n517 = case shown="\"Take LDA data\"" w909 {
                  tunnel: w905 -> [_ w913]
                  tunnel: [string[] [] w912] -> w901
                  frame "No LDA data" {
                  }
                  frame "Take LDA data" {
                    n518 = global read "Meas_global.vi" "Synchronise with LDA"() -> (w918:bool)
                    n519 = global read "Meas_global.vi" "Ch & spans"() -> (w921:T25[])
                    n520 = global read "LDA_meas_global_1.vi" "Probe Configuration"() -> (w911:string)
                    n521 = Array Size(array=w921) -> (size(s)=w920:i32)
                    n522 = Greater Than 0?(x=w920) -> (x > 0?=w919:bool)
                    n523 = Compound Arithmetic op=AND(w918, w913, w919) -> (w917:bool)
                    n524 = Select(t="Synchronised with LDA", s=w917, f="") -> (s? t:f=w914:string)
                    n525 = Build Array(w911, w914) -> (w912:string[])
                  }
                }
                n526 = Compound Arithmetic op=AND(w905, w908) -> (w902:bool)
                n527 = Select(t="Continuous Time Trace", s=w902, f="") -> (s? t:f=w900:string)
                n528 = Build Array (concatenate)(w901, w900) -> (w899:string[])
                n529 = Build Array(w899) -> (w898:string[][])
                n530 = Transpose 2D Array(2D array=w898) -> (transposed array=w897:string[][])
                n531 = local write "BSA Diagnostic info"(w897) -> ()
              }
            }
          }
        }
      }
      frame #18 {
        n532 = local read "File"() -> (w939:T9)
        n533 = Equal?(x=Setup."Run Program" ("setup"), y=w940) -> (x = y?=w937:bool)
        n534 = Not Equal?(x=w939, y=Save_Data."Save No Data" ("File")) -> (x != y?=w938:bool)
        n535 = global read "Meas_global.vi" "Repeat Measurement?"() -> (w922:bool)
        n536 = Compound Arithmetic op=AND(invert w922, w937, w938) -> (w936:bool)
        n537 = Get Date/Time In Seconds() -> (seconds since 1Jan1904=w933:timestamp)
        n538 = To Double Precision Float(number=w933) -> (double precision float=w925:dbl)
        n539 = local read "Setup filename"() -> (w934:string)
        n540 = global read "Trav_pos_global.vi" "Meas Setup Number"() -> (w931:i32)
        n541 = global read "Meas_global.vi" "Board type"() -> (w929:T13)
        n542 = Greater Than 0?(x=w931) -> (x > 0?=w927:bool)
        n543 = Equal?(x=w929, y=Board_Types."Server Channels" ("Board type")) -> (x = y?=w928:bool)
        n544 = And(x=w927, y=w928) -> (x .and. y?=w926:bool)
        n545 = case shown="True" w926 {
          tunnel: w925 -> [_ w944]
          tunnel: [w941 w942] -> w924
          tunnel: w923 -> [w941 _]
          frame False {
          }
          frame True {
            n546 = global read "Trav_pos_global.vi" "Current Row"() -> (w947:T16)
            n547 = Unbundle By Name(w947) -> ("Averaging time (min)"=w945:dbl)
            n548 = Multiply(x=60.0 ("y"), y=w945) -> (x*y=w943:dbl)
            n549 = Subtract(x=w944, y=w943) -> (x-y=w942:dbl)
          }
        }
        n550 = case shown="True" w936 {
          tunnel: w939 -> [_ _]
          tunnel: w925 -> [w950 w1002]
          tunnel: w934 -> [w949 w1001]
          tunnel: w924 -> [w948 w1000]
          frame True {
            n551 = stacked-sequence {
              seq-local: [_ w954 _ _ _] -> [_ _ w960 _ _]
              seq-local: [_ _ _ w973 _] -> [_ _ _ _ w993]
              tunnel: w950 -> [w953 _ _ _ _]
              tunnel: w949 -> [w952 _ _ _ _]
              tunnel: w948 -> [w951 _ _ _ _]
              frame #0 {
                n552 = call "Write_Results_file.vi"("Experiment start time"=w951, "Experiment End time"=w953, "Setup filename"=w952) -> ()  [unwired: 4 out]
              }
              frame #1 {
                n553 = global read "Meas_global.vi" "Second Graph"() -> (w958:T3)
                n554 = global read "Meas_global.vi" "First Graph"() -> (w959:T3)
                n555 = Unbundle By Name(w958) -> ("Save graph"=w956:u16)
                n556 = Unbundle By Name(w959) -> ("Save graph"=w957:u16)
                n557 = Add(x=w957, y=w956) -> (x+y=w955:u16)
                n558 = Not Equal To 0?(x=w955) -> (x != 0?=w954:bool)
              }
              frame #2 {
                n559 = case shown="True" w960 {
                  frame False {
                  }
                  frame True {
                    n560 = stacked-sequence {
                      tunnel: "Show Smoth" -> [w964 w965]
                      frame #0 {
                        n561 = local read "First plot"() -> (w963:cluster{"Xo":dbl, "Delta X":dbl, dbl[]}[])
                        n562 = local read "2nd plot"() -> (w962:cluster{"Xo":dbl, "Delta X":dbl, dbl[]}[])
                        n563 = call "Save_plot_routine.vi"("Show Smooth"=w964, "First Plot data"=w963, "Second Plot data"=w962) -> ()  [unwired: 1 in, 3 out]
                      }
                      frame #1 {
                        n564 = case shown="True" w965 {
                          frame False {
                          }
                          frame True {
                            n565 = Open VI Reference(vi path="Measurement.vi") -> (vi reference=w971:refnum<vi>, error out=w967:errorcluster)  [unwired: 1 in, 4 out]
                            n566 = local write "Show Smoth"(FALSE ("Show Smoth")) -> ()
                            n567 = property class="VI"(reference=w971, error in=w967, "Front Panel Window:Is Frontmost"=TRUE) -> (reference out=w969:refnum<vi>, error out=w968:errorcluster)
                            n568 = Close Reference(reference=w969, error in (no error)=w968) -> ()  [unwired: 1 out]
                          }
                        }
                      }
                    }
                  }
                }
              }
              frame #3 {
                w978 = FALSE  # Empty list
                n569 = global read "Meas_global.vi" "Raw data file"() -> (w977:path)
                n570 = global read "Trav_pos_global.vi" "Top level setup filename"() -> (w975:path)
                n571 = global read "Meas_global.vi" "Start Time of experiment"() -> (w974:dbl)
                n572 = Strip Path(path=w977) -> (stripped path=w973:path)  [unwired: 1 out]
                n573 = Empty String/Path?(string/path=w975) -> (empty?=w976:bool)
                n574 = case shown="False" w976 {
                  tunnel: w975 -> [w992 _]
                  tunnel: w973 -> [w990 _]
                  tunnel: w974 -> [w988 _]
                  frame False {
                    n575 = call "Sec_to_date_filename.vi"("seconds"=w988) -> ("Day"=w987:string, "Time"=w986:string)  [unwired: 2 out]
                    n576 = Format Into String(format string="Cmd_%s_%s.xls", w987, w986) -> (resulting string=w984:string)  [unwired: 2 in, 1 out]
                    n577 = call "Fast_string_Replace.vi"("Replace match with:"="-", "Input String"=w984, "regular expression"=":") -> ("Output String"=w981:string)  [unwired: 2 out]
                    n578 = call "Fast_string_Replace.vi"("Replace match with:"="", "Input String"=w981, "regular expression"=" ") -> ("Output String"=w979:string)  [unwired: 2 out]
                    n579 = Build Path(base path=w990, name or relative path=w979) -> (appended path=w989:path)
                    n580 = Copy(10:w989, 11:w992) -> ()  [unwired: 1 in, 5 out]
                  }
                  frame True {
                  }
                }
                n581 = call "Remember_RD_Folders.vi"("Empty list"=w978, "Folders to Remember"=w973) -> ()  [unwired: 1 out]
              }
              frame #4 {
                n582 = global read "Meas_global.vi" "LDA data"() -> (w994:enum16{"No LDA data", "Take LDA data"})
                n583 = case shown="\"Take LDA data\"" w994 {
                  tunnel: w993 -> [_ w995]
                  frame "No LDA data" {
                  }
                  frame "Take LDA data" {
                    w997 = "LDA_Probe_Orientation.txt" ("name or relative path")
                    n584 = global read "Constants_global.vi" "General folder"() -> (w999:path)
                    n585 = Build Path(base path=w999, name or relative path=w997) -> (appended path=w998:path)
                    n586 = Build Path(base path=w995, name or relative path=w997) -> (appended path=w996:path)
                    n587 = Copy(10:w996, 11:w998) -> ()  [unwired: 1 in, 5 out]
                  }
                }
              }
            }
          }
          frame False {
            n588 = global read "Meas_global.vi" "Raw data option"() -> (w1003:enum16{"Save raw data", "Raw data not saved"})
            n589 = case shown="\"Save raw data\"" w1003 {
              tunnel: w1000 -> [w1006 _]
              tunnel: w1002 -> [w1005 _]
              tunnel: w1001 -> [w1004 _]
              frame "Save raw data" {
                n590 = stacked-sequence {
                  tunnel: w1006 -> [_ w1015]
                  tunnel: w1005 -> [_ w1014]
                  tunnel: w1004 -> [_ w1012]
                  frame #0 {
                    n591 = global read "Meas_global.vi" "Current Block No"() -> (w1007:i32)
                    n592 = global write "Meas_global.vi" "Requested No of blocks"(w1007) -> ()
                  }
                  frame #1 {
                    n593 = call "Create_Raw_data_file.vi"("No of averages"=1, "End time"=w1014, "Start time"=w1015, "Setup filename"=w1012) -> ("Values"=w1010:string[][], "Column headers"=w1011:string[])  [unwired: 2 out]
                    n594 = Index Array(array=w1010, index (row)=0) -> (element=w1008:string[])  [unwired: 1 in]
                    n595 = global write "Dynamic_call_global.ph.vi" "Plug in values"(w1008) -> ()
                    n596 = global write "Dynamic_call_global.ph.vi" "Plug in titles"(w1011) -> ()
                  }
                }
              }
              frame "Raw data not saved" {
              }
            }
          }
        }
      }
      frame #19 {
        n597 = stacked-sequence {
          seq-local: [w1022 _] -> [_ w1031]
          seq-local: [w1018 _] -> [_ w1030]
          tunnel: w1016 -> [w1029 _]
          frame #0 {
            n598 = global read "Meas_global.vi" "Raw data file"() -> (w1020:path)
            n599 = global read "Meas_global.vi" "Raw data option"() -> (w1028:enum16{"Save raw data", "Raw data not saved"})
            n600 = Equal?(x=Setup."Run Program" ("setup"), y=w1029) -> (x = y?=w1024:bool)
            n601 = Strip Path(path=w1020) -> (stripped path=w1019:path)  [unwired: 1 out]
            n602 = Equal?(x=w1028, y=enum16{"Save raw data", "Raw data not saved"}."Save raw data" ("Raw data option")) -> (x = y?=w1023:bool)
            n603 = Build Path(base path=w1019, name or relative path="VI_History.xls") -> (appended path=w1018:path)
            n604 = call "Does_file_exist_(simple).vi"("Pathname"=w1018) -> ("exists?"=w1026:bool)
            n605 = Not(x=w1026) -> (.not. x?=w1025:bool)
            n606 = Compound Arithmetic op=AND(w1025, w1024, w1023) -> (w1022:bool)
          }
          frame #1 {
            n607 = case shown="True" w1031 {
              tunnel: w1030 -> [_ w1038]
              frame False {
              }
              frame True {
                w1032 = FALSE  # Lock File
                n608 = global read "Meas_global.vi" "Prog's last revision date"() -> (w1035:u32)
                n609 = Get Date/Time String(date format (0)=enum16{"short", "long", "abbreviated"}."abbreviated", seconds (now)=w1035) -> (date string=w1034:string)  [unwired: 2 out]
                n610 = call "Characters_to_string.vi"("Characters to write"=w1034, "Label for characters"="Prog's last revision date") -> ("Output string"=w1040:string)
                n611 = call "Date_and_Time_to_string.vi"() -> ("Date and time (spreadsheet)"=w1041:string)
                n612 = call "Get_mod_dates.vi"() -> ("error out"=w1039:errorcluster, "Output string"=w1033:string)  [unwired: 1 in, 3 out]
                n613 = call "EnFlo_Error_Handler.vi"("error in (no error)"=w1039) -> ()  [unwired: 2 in, 3 out]
                n614 = Concatenate Strings(w1041, w1040, w1033) -> (w1037:string)
                n615 = call "Write_Characters_To_File.vi"("file path (dialog if empty)"=w1038, "character string"=w1037, "Lock File"=w1032) -> ()  [unwired: 2 in, 4 out]
              }
            }
          }
        }
      }
      frame #20 {
        w1045 = FALSE ("Remote control")
        n616 = local read "Correlate?"() -> (w1047:T6)
        n617 = case shown="\"Run Program\"" w1044 {
          tunnel: w1044 -> [w1051 _ _ _]
          tunnel: [w1051 w1068 w1069 w1070] -> w1043
          frame "Run Program" {
            n618 = global read "Meas_global.vi" "Velocity Cluster Array"() -> (w1050:T26[])
            n619 = Array Size(array=w1050) -> (size(s)=w1049:i32)
            n620 = Decrement(x=w1049) -> (x-1=w1048:i32)
            n621 = while {
              tunnel: w1050 -> [w1066] mode=indexing
              tunnel: w1048 -> [w1057]
              i -> [w1058]
              stop <- w1055 continue-if-true
              w1063 = "Pitot ("
              n622 = Unbundle By Name(w1066) -> ("U"=w1052:dbl, "Name"=w1062:string)
              n623 = String Length(string=w1063) -> (length=w1065:i32)
              n624 = String Subset(string=w1062, length (rest)=w1065) -> (substring=w1064:string)  [unwired: 1 out]
              n625 = Equal?(x=w1064, y=w1063) -> (x = y?=w1059:bool)
              n626 = call "Match_Pat_Case_In.vi"("String to match"="ref", "String"=w1062) -> ("offset past match"=w1060:i32)  [unwired: 1 in, 3 out]
              n627 = Greater Or Equal To 0?(x=w1060) -> (x >= 0?=w1054:bool)
              n628 = Less?(x=w1058, y=w1057) -> (x < y?=w1056:bool)
              n629 = And(x=w1054, y=w1059) -> (x .and. y?=w1053:bool)
              n630 = case shown="True" w1053 {
                tunnel: w1052 -> [_ w1067]
                frame False {
                }
                frame True {
                  n631 = call "Log_Reference_Velocity.vi"("Measured Velocity"=w1067) -> ()  [unwired: 1 out]
                }
              }
              n632 = Compound Arithmetic op=AND(invert w1053, w1056) -> (w1055:bool)
            }
          }
          frame "Show Setup" {
            w1068 = Setup."Run Program"  # setup
          }
          frame "Save Current Setup" {
            w1069 = Setup."Run Program"  # setup
          }
          frame "Setup Front Panel" {
            w1070 = Setup."Run Program"  # setup
          }
        }
        n633 = case shown="\"Correlate without activating panel\"" w1047 {
          tunnel: [T6."Cross correlation off" T6."Correlate without activating panel" T6."Correlate without activating panel"] -> w1046
          frame "Cross correlation off" {
          }
          frame "Show correlation panel" {
          }
          frame "Correlate without activating panel" {
          }
        }
        n634 = local write "Correlate?"(w1046) -> ()
        n635 = global write "Meas_global.vi" "Remote control"(w1045) -> ()
        n636 = global write "Dynamic_call_global.ph.vi" "Acquisition Interlock"(w1045) -> ()
        n637 = call "Program_Active.vi"() -> ()  [unwired: 1 in]
        n638 = local write "setup"(w1043) -> ()
      }
      frame #21 {
        w1078 = FALSE  # Dialog Box (T)
        n639 = global read "Meas_global.vi" "Over/Under string"() -> (w1076:string)
        n640 = Empty String/Path?(string/path=w1076) -> (empty?=w1075:bool)
        n641 = Not(x=w1075) -> (.not. x?=w1074:bool)
        n642 = Bundle By Name(cluster=errorcluster {"status"=FALSE, "code"=0, "source"=""} ("error in (no error)"), "source"=w1076, "status"=w1074) -> (w1079:errorcluster)
        n643 = call "EnFlo_Error_Handler.vi"("error in (no error)"=w1079, "Error Type"="Signal Clipping", "Dialog Box (T)"=w1078) -> ()  [unwired: 3 out]
      }
      frame #22 {
        w1083 = string[] [] ("Per Block Plug Ins Extra")
        n644 = Empty String/Path?(string/path=w1087) -> (empty?=w1086:bool)
        n645 = global read "Dynamic_call_global.ph.vi" "Final Plug Ins"() -> (w1088:string[])
        n646 = case shown="True" w1086 {
          tunnel: w1087 -> [w1100 _]
          frame False {
            n647 = local read "Comments"() -> (w1099:string)
            n648 = call "Fast_string_Replace.vi"("Replace match with:"="", "Input String"=w1099, "regular expression"=w1100) -> ("Output String"=w1098:string)  [unwired: 2 out]
            n649 = local write "Comments"(w1098) -> ()
          }
          frame True {
          }
        }
        n650 = call "Plug_in_Directories.vi"() -> ("Final"=w1084:path)  [unwired: 3 out]
        n651 = for {
          tunnel: w1088 -> [w1103] mode=indexing
          tunnel: w1084 -> [w1102]
          w1106 = FALSE  # Dialog Box (T)
          n652 = Build Path(base path=w1102, name or relative path=w1103) -> (appended path=w1101:path)
          n653 = global read "Dynamic_call_global.ph.vi" "Plug in"() -> (w1111:refnum<vi>)
          n654 = Open VI Reference(type specifier VI Refnum (for type only)=w1111, vi path=w1101) -> (vi reference=w1110:refnum<vi>, error out=w1109:errorcluster)  [unwired: 2 in, 2 out]
          n655 = call-by-ref "?"(reference=w1110, error in=w1109) -> (reference out=w1107:refnum<vi>, error out=w1108:errorcluster)  [unwired: 6 in, 2 out]
          n656 = Close Reference(reference=w1107, error in (no error)=w1108) -> (error out=w1104:errorcluster)
          n657 = call "EnFlo_Error_Handler.vi"("error in (no error)"=w1104, "Error Type"="Running Final Plug In", "Dialog Box (T)"=w1106) -> ()  [unwired: 3 out]
        }
        n658 = global read "Meas_global.vi" "Repeat Measurement?"() -> (w1085:bool)
        n659 = case shown="False" w1085 {
          tunnel: w1082 -> [_ w1096]
          tunnel: [FALSE w1091] -> w1081
          frame False {
            n660 = global write "Trav_pos_global.vi" "Present Probe Positions"(T7 [] ("Present Probe Positions")) -> ()
          }
          frame True {
            n661 = global read "Meas_global.vi" "Post Process"() -> (w1094:T5)
            n662 = Equal To 0?(x=w1096) -> (x = 0?=w1092:bool)
            n663 = Equal?(x=w1094, y=Post_Process."Post Process Raw Data File" ("Post Process")) -> (x = y?=w1093:bool)
            n664 = And(x=w1093, y=w1092) -> (x .and. y?=w1091:bool)
          }
        }
        n665 = global write "Dynamic_call_global.ph.vi" "Per Block Plug Ins Extra"(w1083) -> ()
        n666 = global write "Dynamic_call_global.ph.vi" "Initial Plug Ins Extra"(w1083) -> ()
      }
      frame #23 {
        n667 = global read "Meas_global.vi" "Post Process"() -> (w1118:T5)
        n668 = local read "stop"() -> (w1124:bool)
        n669 = Equal?(x=w1119, y=Setup."Run Program" ("setup")) -> (x = y?=w1115:bool)
        n670 = Equal?(x=w1118, y=Post_Process."Take New Data" ("Post Process")) -> (x = y?=w1116:bool)
        n671 = And(x=w1115, y=w1116) -> (x .and. y?=w1114:bool)
        n672 = case shown="False" w1124 {
          tunnel: [Multi_Run_Status."Continue" ("Status Out") Multi_Run_Status."Terminate Run" ("Status Out")] -> w1122
          frame False {
          }
          frame True {
            n673 = local write "stop"(FALSE) -> ()
          }
        }
        n674 = case shown="True" w1114 {
          tunnel: w1122 -> [w1125 w1128]
          tunnel: [w1125 w1130] -> w1121
          frame False {
          }
          frame True {
            n675 = local read "Raw data file"() -> (w1129:path)
            n676 = Path to Array of Strings(0:w1129) -> (2:w1131:string[])  [unwired: 1 out]
            n677 = Index Array(array=w1131, index=0 ("Index")) -> (element=w1127:string)
            n678 = Build Array(w1127) -> (w1126:string[])
            n679 = for {
              tunnel: w1126 -> [w1135] mode=indexing
              shift-right: [w1133] -> w1130
              shift-left: w1128 -> [w1134]
              n680 = call "Warn_on_low_HD_space.vi"("Status In"=w1134, "HD name"=w1135) -> ("Status Out"=w1133:T4)  [unwired: 6 out]
            }
          }
        }
        "Status Out" <- w1121
        n681 = global write "Trav_pos_global.vi" "Dummy Measurement?"(FALSE ("Dummy Measurement?")) -> ()
        n682 = global write "Plug_in_data_global.vi" "Server Channels to log"(string[] [] ("Server Channels to log")) -> ()
        n683 = global write "Meas_global.vi" "Extra Comments"("") -> ()
      }
    }
  }
